vi "Autonomous Independent.vi"   [LabVIEW 2015]
doc: "This VI is called when autonomous begins, and will automatically be terminated when autonomous ends. You can carry out timed or sensor driven robot movement independently without needing to return to the caller."
uses:
  <vilib>/Rock Robotics/WPI/Solenoid/WPI_SolenoidValue.ctl
  <vilib>/Rock Robotics/WPI/Utilities/WPI_GetSetVariantRefNum.vi
  <vilib>/Rock Robotics/Network Tables/NT Write Numeric Array.vi
  <vilib>/Rock Robotics/Network Tables/NT Read String.vi
  <vilib>/Rock Robotics/WPI/Solenoid/WPI_SolenoidSetEnum.vi
  <vilib>/Rock Robotics/WPI/RobotDrive/WPI_RobotDriveArcadeDrive_Standard(NoSaturation).vi
panel:
  # "Be sure to right-click and choose Data Operations>>Make Current Value default if you want to save the array values with the VI"
types:
  T1 = typedef "WPI_JoystickDevRef.ctl" = cluster{"Device":T2}
  T2 = typedef "WPI_JoystickDeviceEnum.ctl" = enum16{"USB 0", "USB 1", "USB 2", "USB 3", "USB 4", "USB 5"}
  T3 = typedef "WPI_SolenoidValue.ctl" = enum16{"Off", "On", "Forward", "Reverse"}
  T4 = typedef "WPI_SolenoidDevRef.ctl" = cluster{"DevStatus":errorcluster, "Pneumatics Control Module":u8, "Forward Solenoid Channel":T5, "Reverse Solenoid Channel":T5}
  T5 = typedef "WPI_SolenoidChannel.ctl" = enum8{"Solenoid 0", "Solenoid 1", "Solenoid 2", "Solenoid 3", "Solenoid 4", "Solenoid 5", "Solenoid 6", "Solenoid 7", "Invalid"}
  T6 = typedef "WPI_RobotDriveDevRef.ctl" = cluster{"DevStatus":errorcluster, "Motors[]":T7[], "Square Inputs":bool, "Max Output":dbl}
  T7 = typedef "WPI_MotorControlDeviceRef.ctl" = cluster{"DeviceStatus":errorcluster, "Type":T8, "PWM":cluster{"PWM Channel":T9, "DeadBand":T10}, "CAN":cluster{"Device Number":u8, "Control Mode":T11, "Semaphore":T12, "Max Vout":dbl, "TalonSRX Control Mode":T13}, "Invert":bool}
  T8 = typedef "WPI_MotorControlType.ctl" = enum16{"PWM", "CAN", "CANTalonSRX"}
  T9 = typedef "FPGA_DIOPWMChannel.ctl" = enum8{"PWM 0", "PWM 1", "PWM 2", "PWM 3", "PWM 4", "PWM 5", "PWM 6", "PWM 7", "PWM 8", "PWM 9", "PWM MXP 0", "PWM MXP 1", "PWM MXP 2", "PWM MXP 3", "PWM MXP 4", "PWM MXP 5", "PWM MXP 6", "PWM MXP 7", "PWM MXP 8", "PWM MXP 9", "Invalid"}
  T10 = typedef "WPI_PWMDeadband.ctl" = cluster{"Name":string, "maxPositivePwm":i32, "minPositivePwm":i32, "centerPwm":i32, "maxNegativePwm":i32, "minNegativePwm":i32, "angularRange":u16}
  T11 = typedef "WPI_CANJaguar_ControlMode.ctl" = enum8{"Percent VBus", "Current", "Speed", "Position", "Voltage"}
  T12 = typedef "Semaphore RefNum" = refnum<k1>
  T13 = typedef "WPI_CANTalonSRX_APIControlMode.ctl" = enum8{"Percent VBus", "Speed", "Position", "Slave", "Unchanged / Invalid", "Voltage Compensation", "Current", "Motion Profile"}
  T14 = typedef "WPI_EncoderDevRef.ctl" = cluster{"DevStatus":errorcluster, "EncoderIndex":T15, "CounterIndex":T16, "DistancePerCount":dbl, "Decoding Type":T17}
  T15 = typedef "FPGA_EncoderIdx.ctl" = enum8{"Enc 0", "Enc 1", "Enc 2", "Enc 3", "Enc 4", "Enc 5", "Enc 6", "Enc 7", "Invalid"}
  T16 = typedef "FPGA_CounterCtrSystemIndex.ctl" = enum8{"Ctr 0", "Ctr 1", "Ctr 2", "Ctr 3", "Ctr 4", "Ctr 5", "Ctr 6", "Ctr 7", "Invalid"}
  T17 = typedef "WPI_EncoderType.ctl" = enum16{"1x", "2x", "4x"}
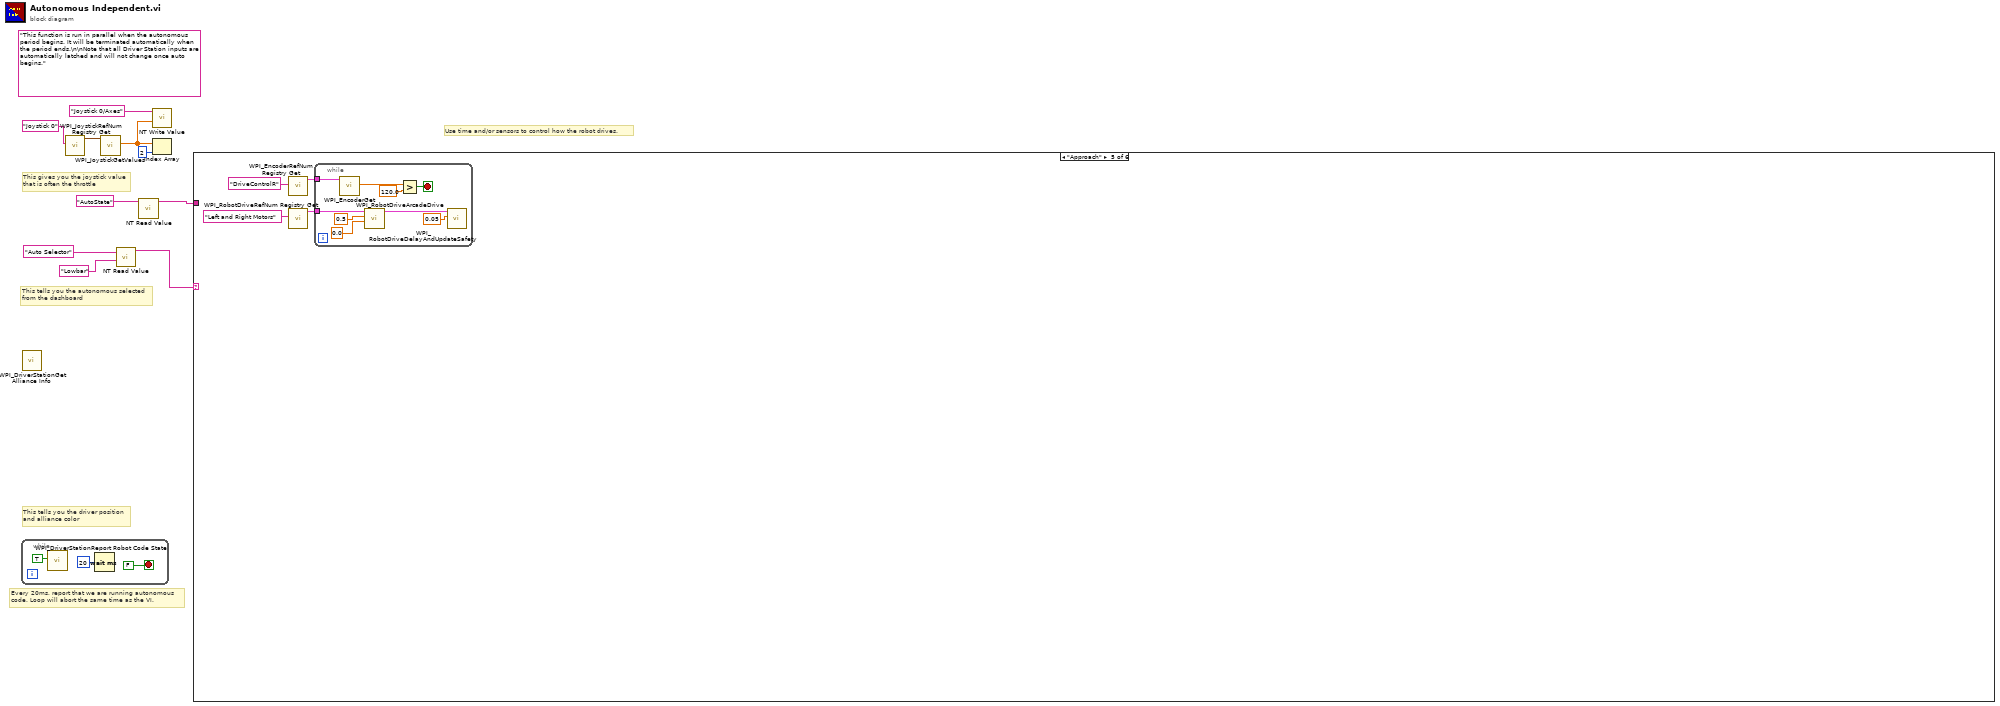
[diagram p0: block diagram]
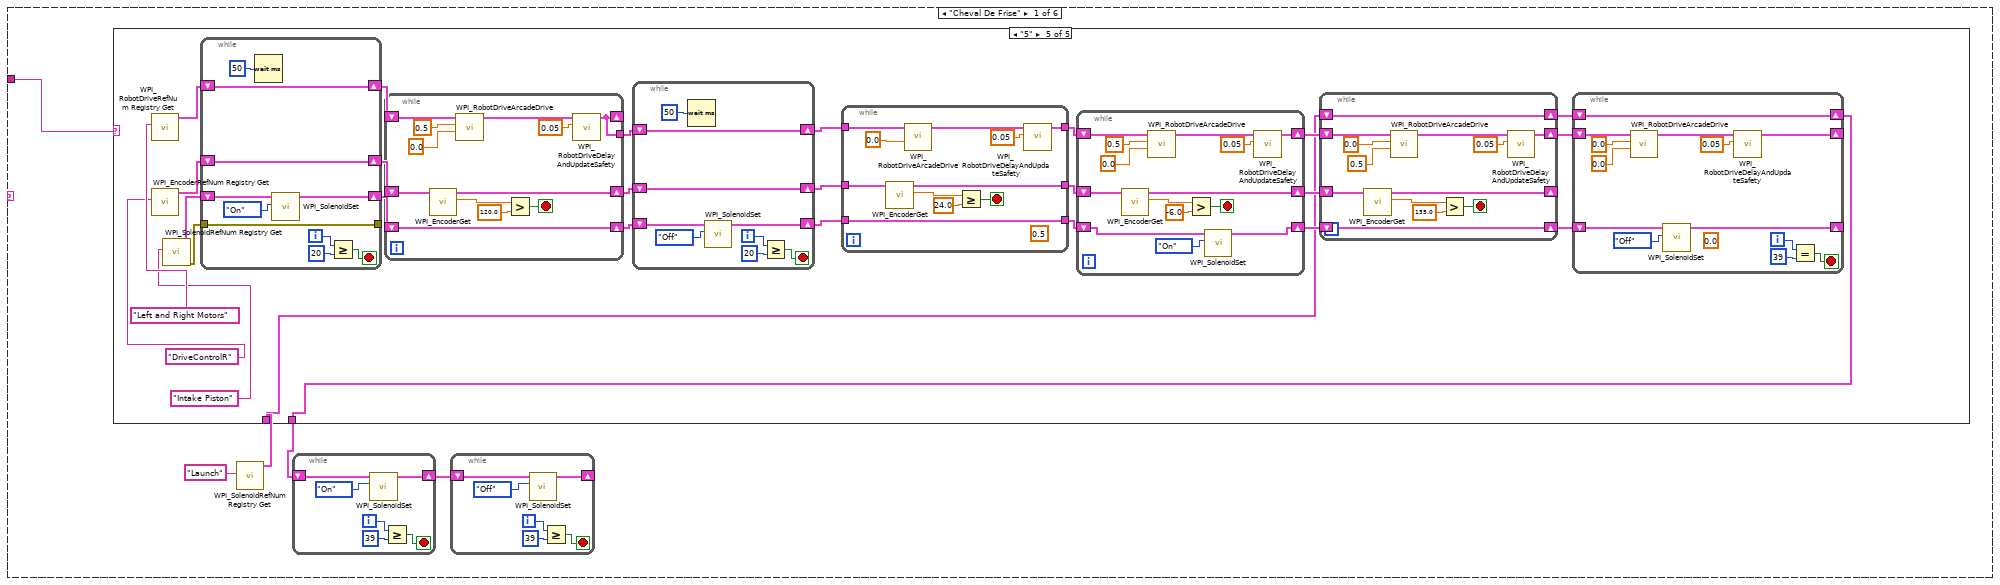
[diagram p2: hidden frame]
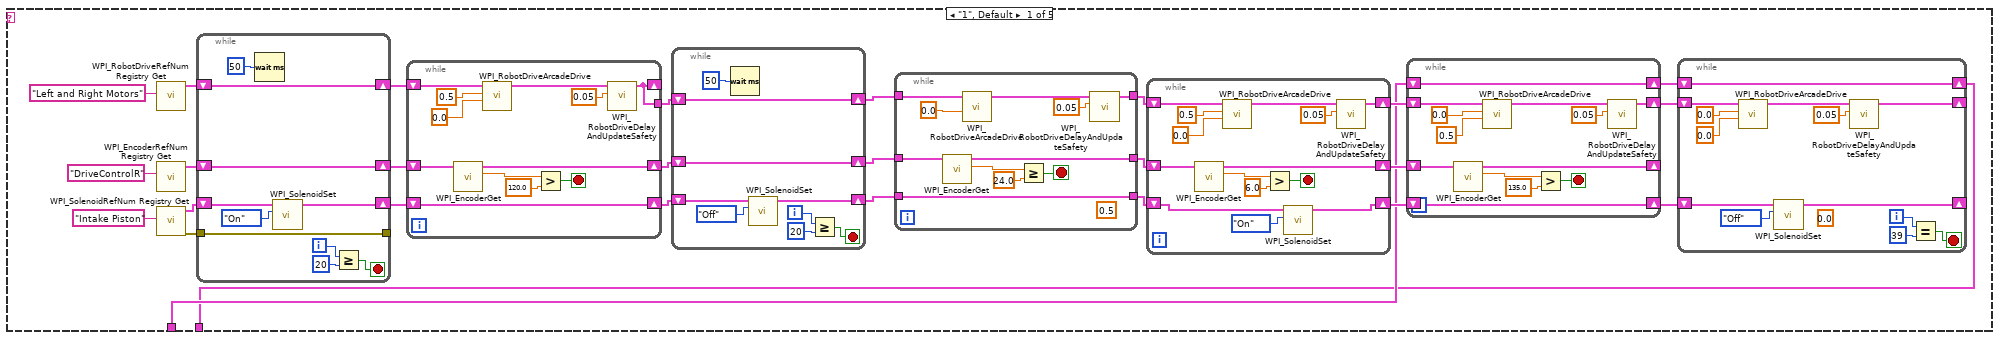
[diagram p3: hidden frame]
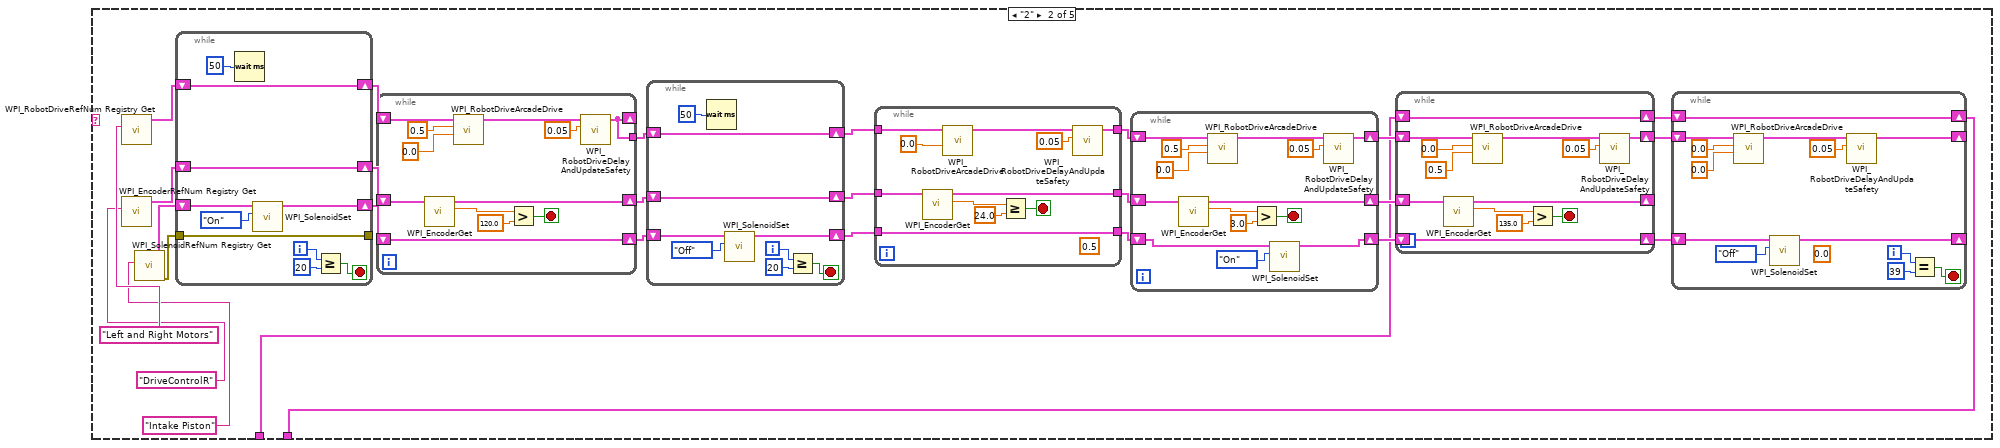
[diagram p4: hidden frame]
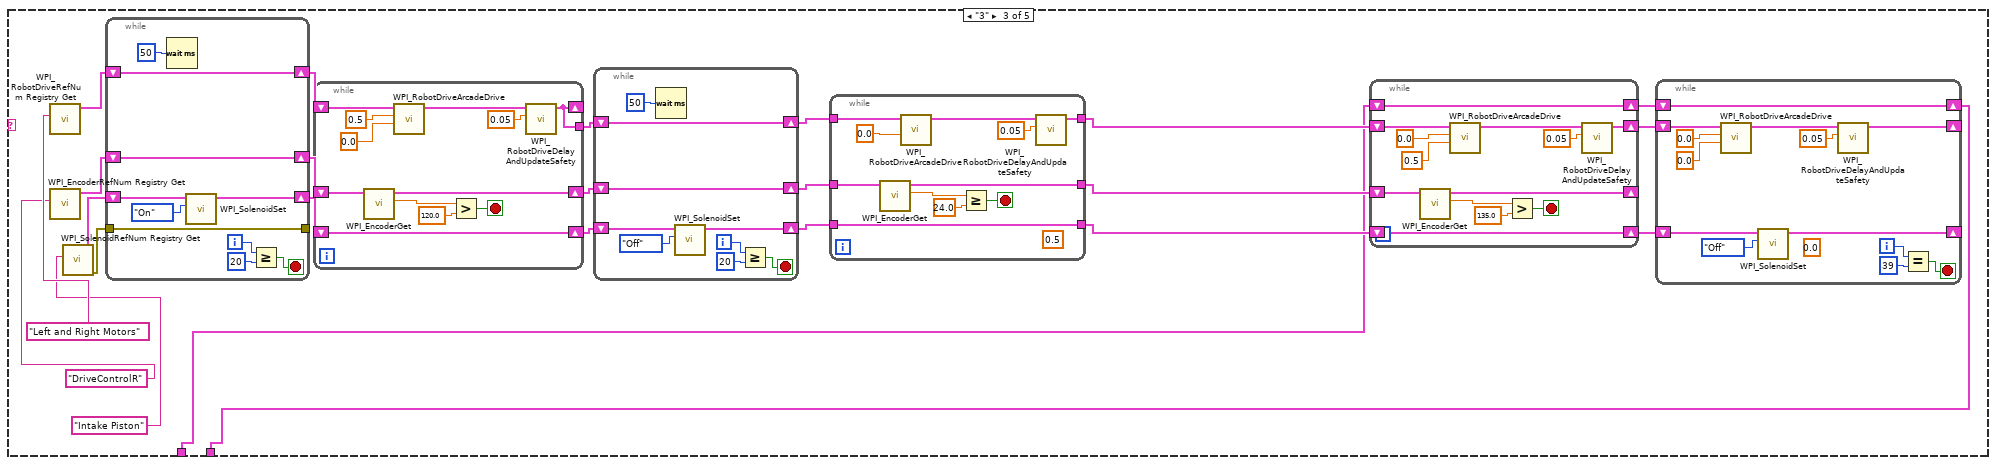
[diagram p5: hidden frame]
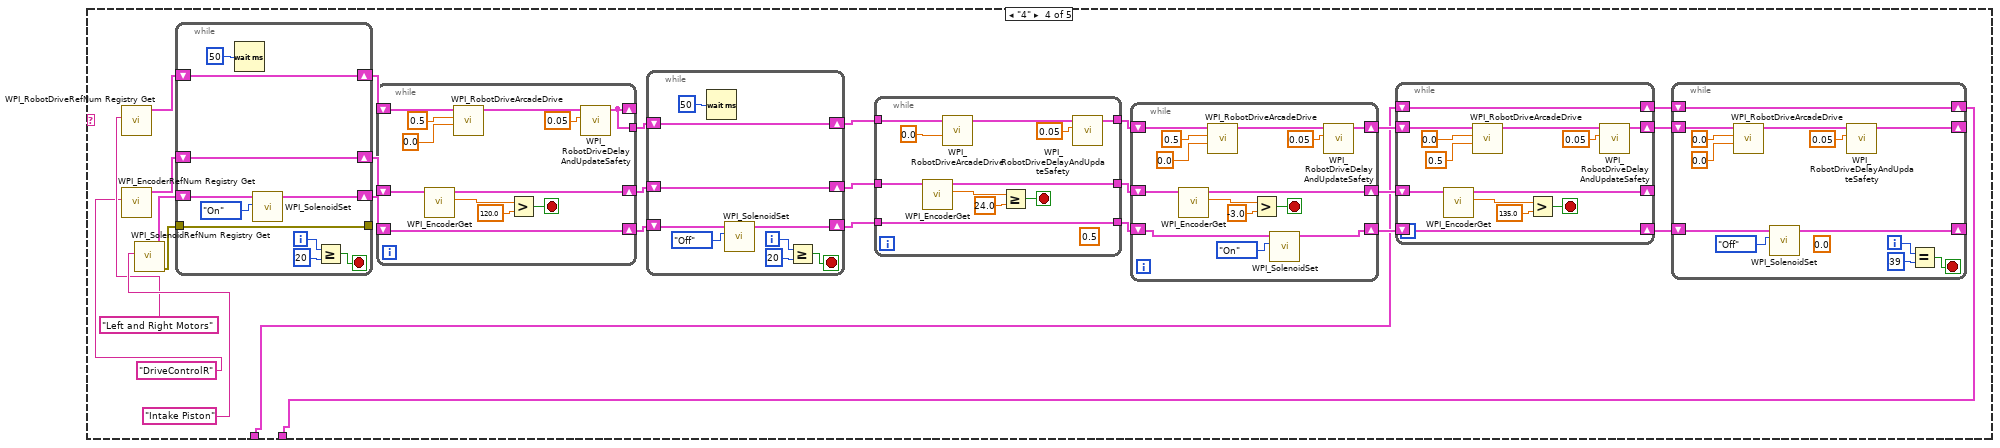
[diagram p6: hidden frame]
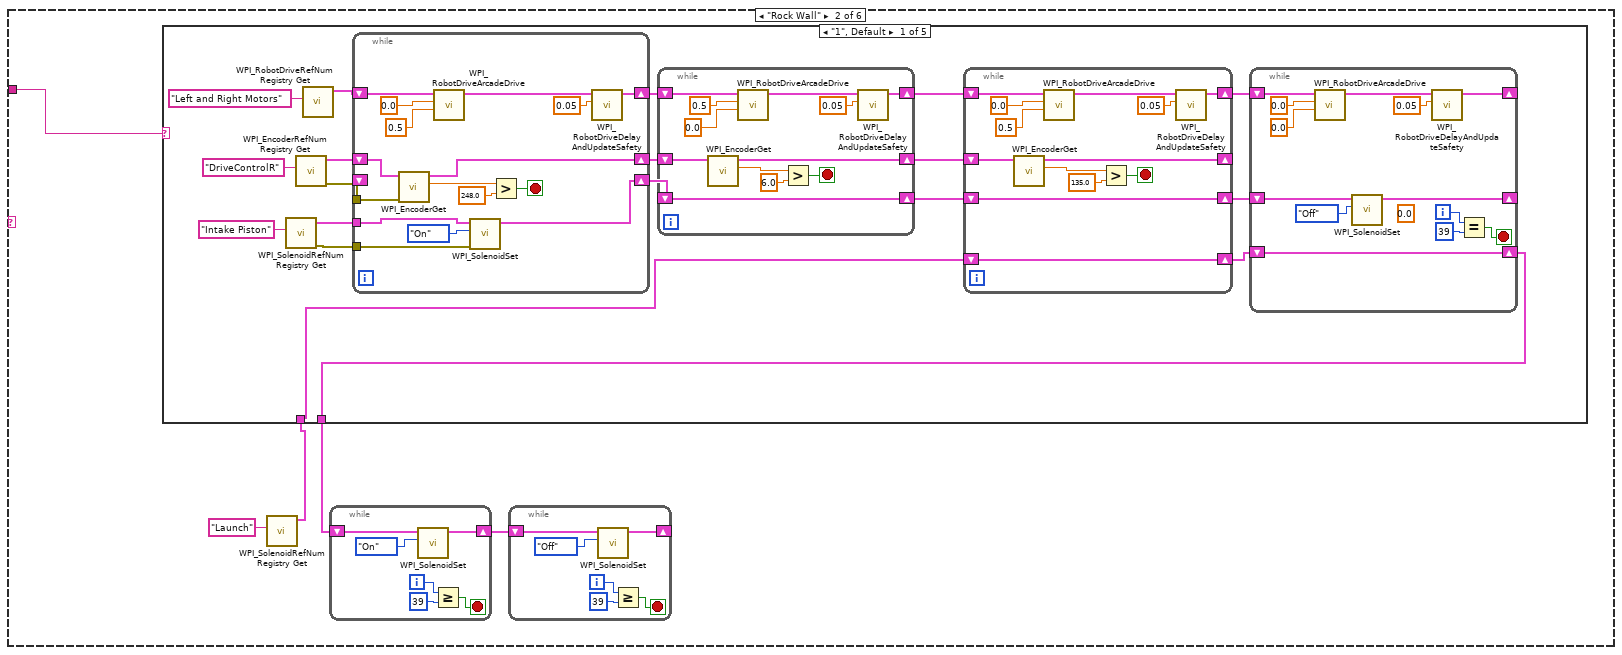
[diagram p7: hidden frame]
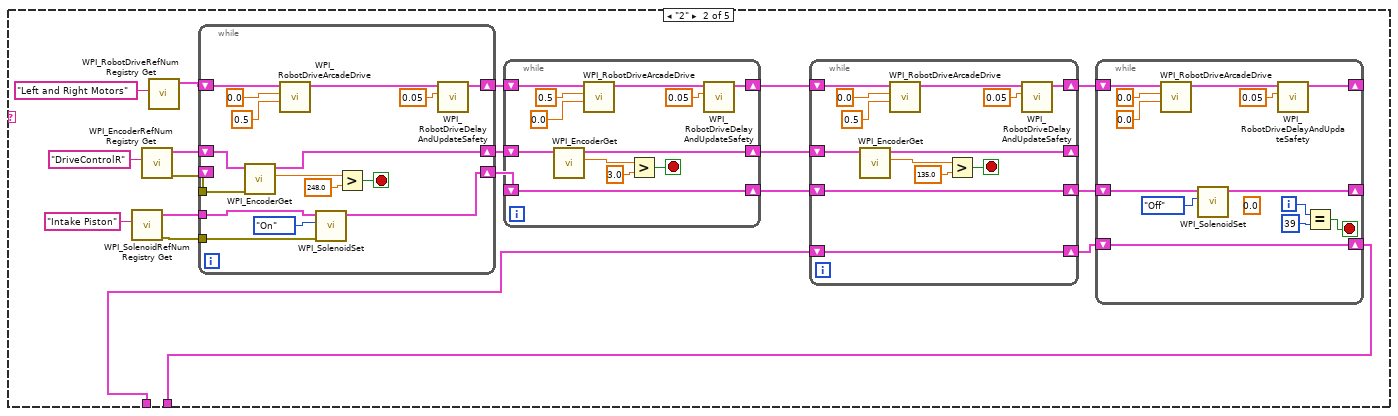
[diagram p8: hidden frame]
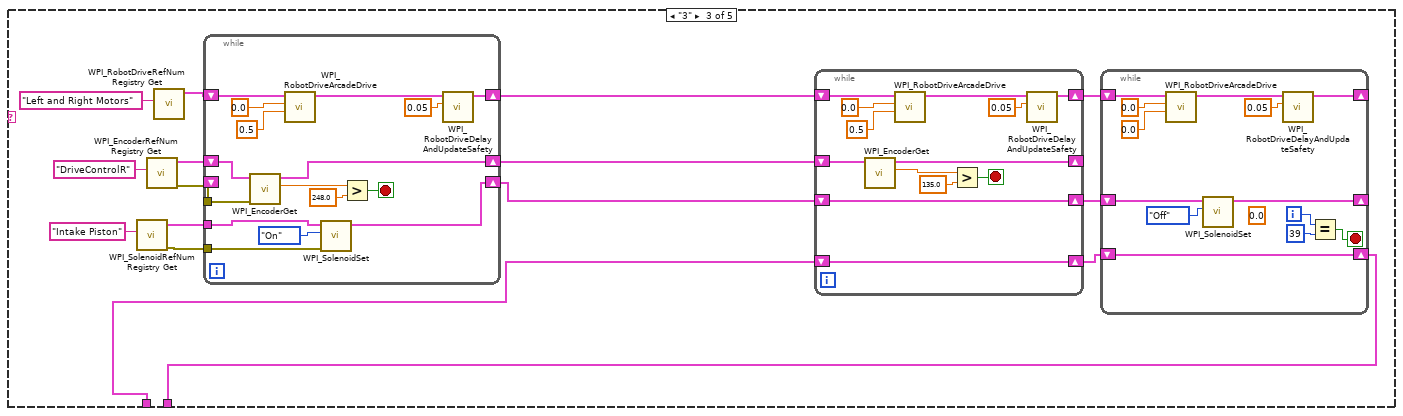
[diagram p9: hidden frame]
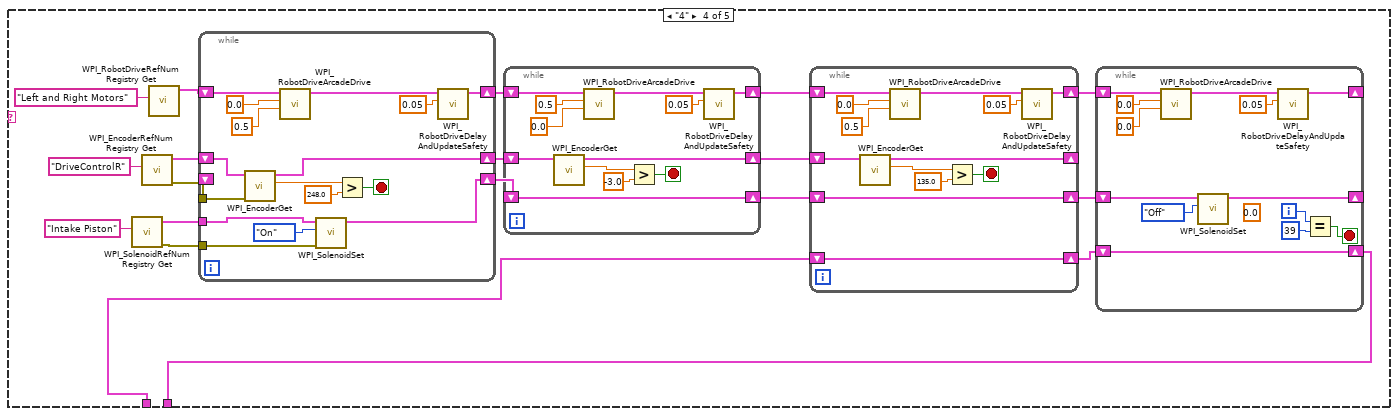
[diagram p10: hidden frame]
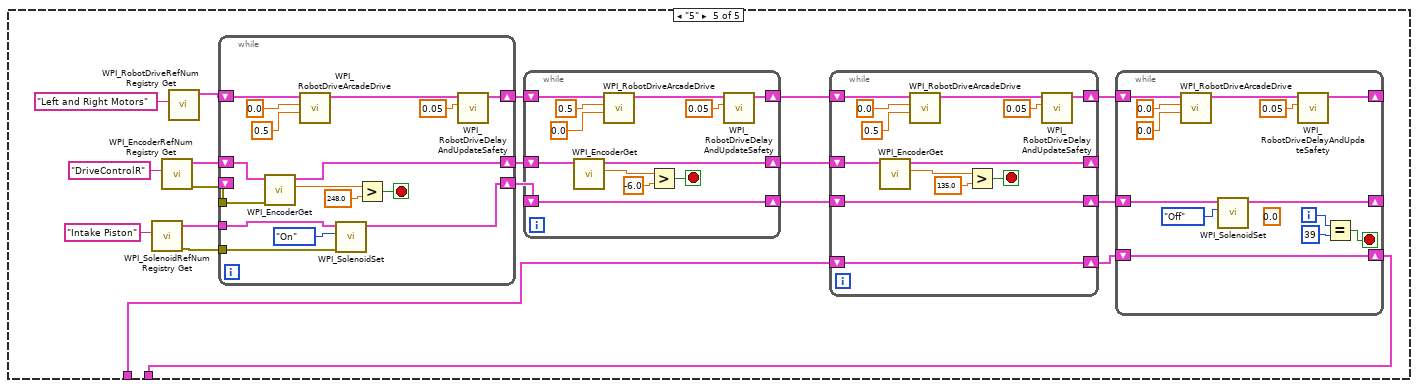
[diagram p11: hidden frame]
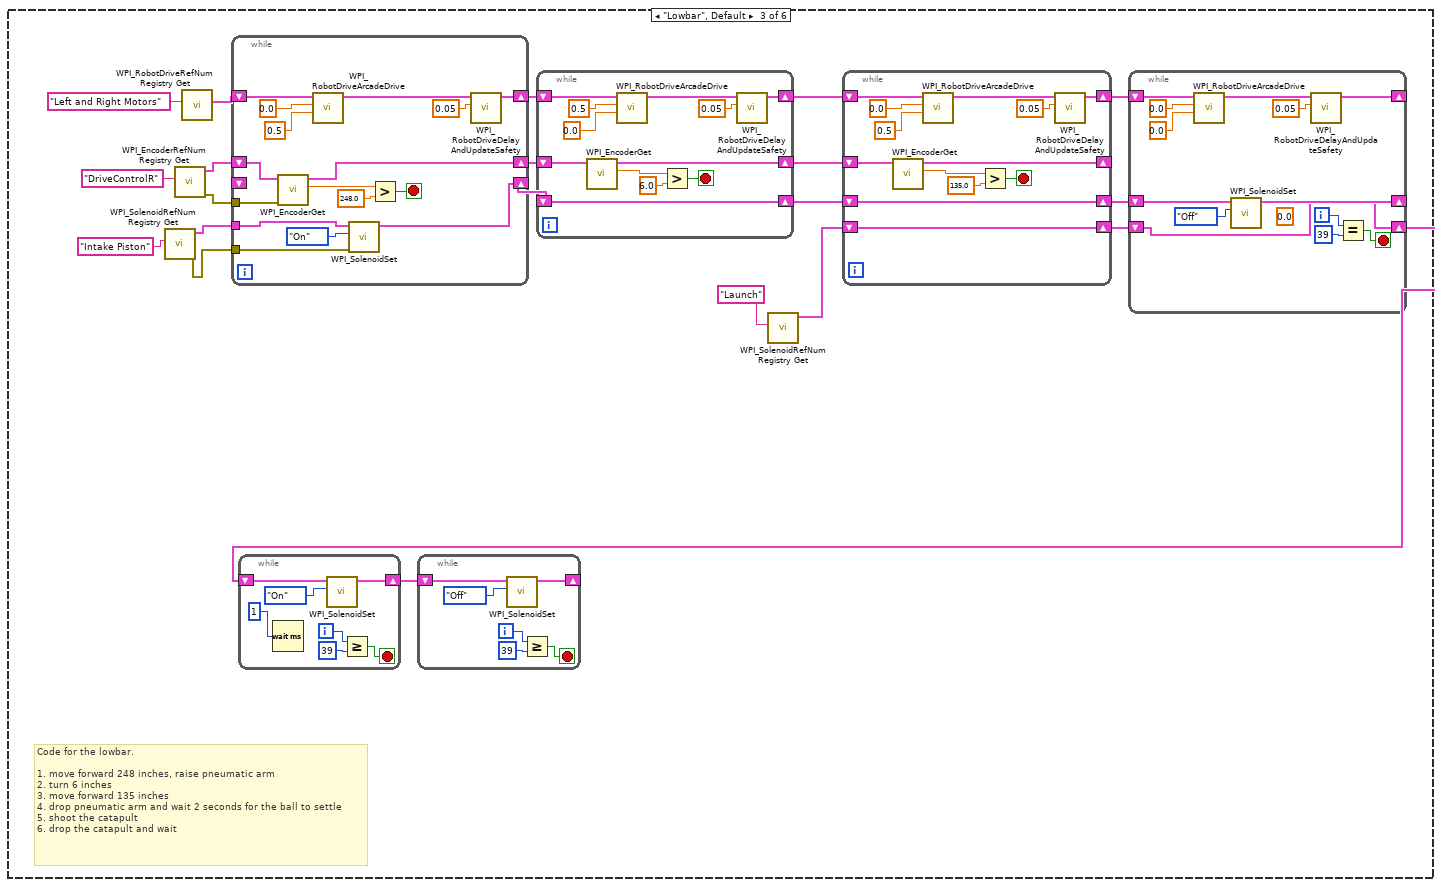
[diagram p12: hidden frame]
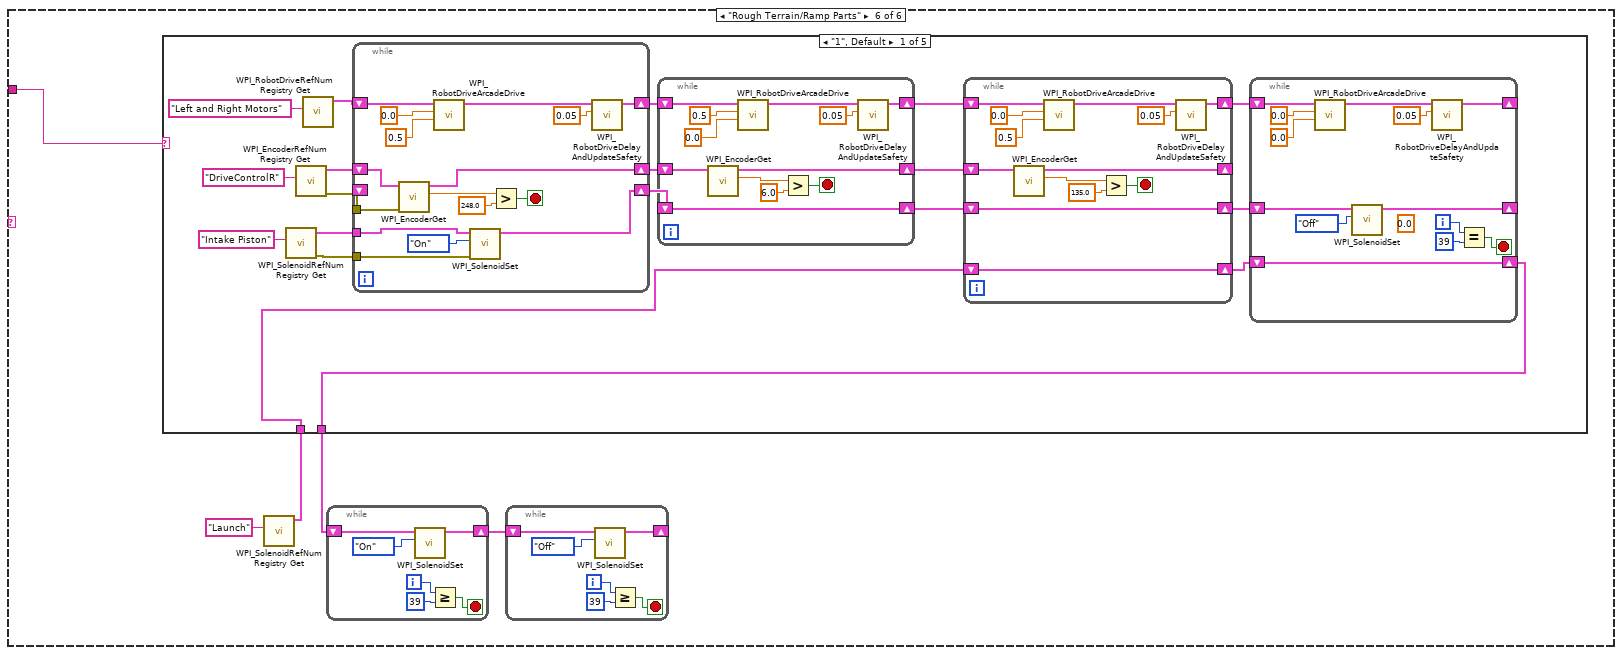
[diagram p14: hidden frame]
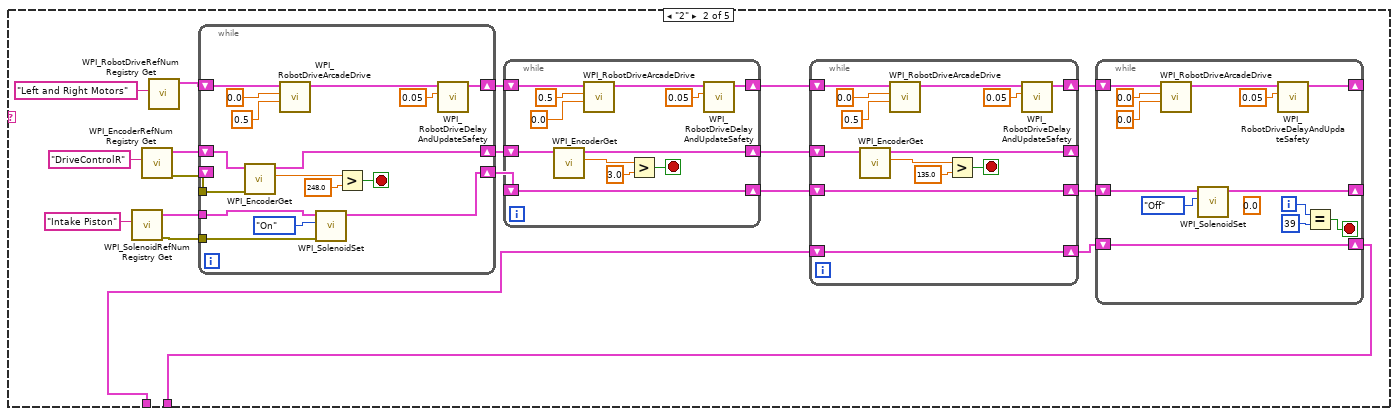
[diagram p15: hidden frame]
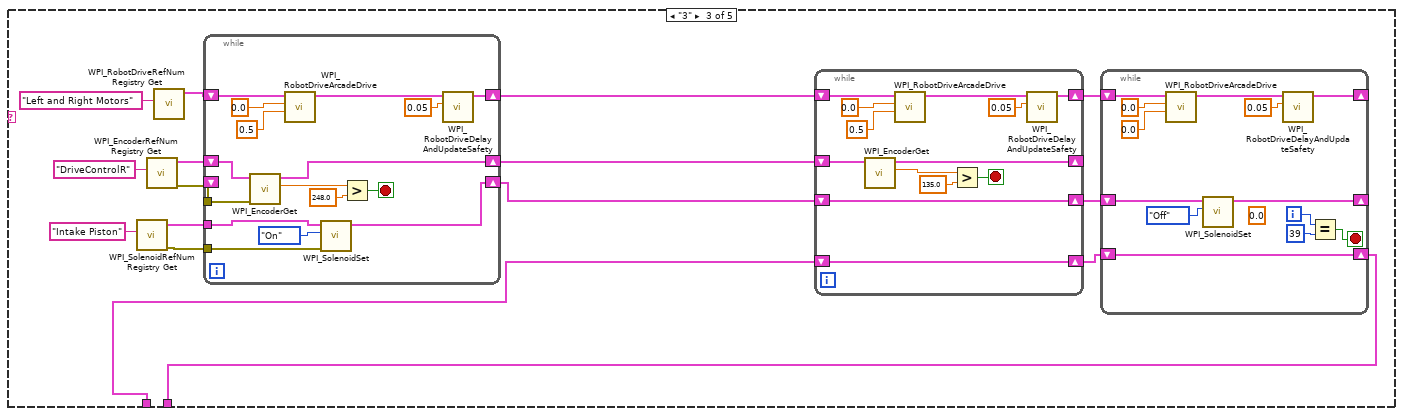
[diagram p16: hidden frame]
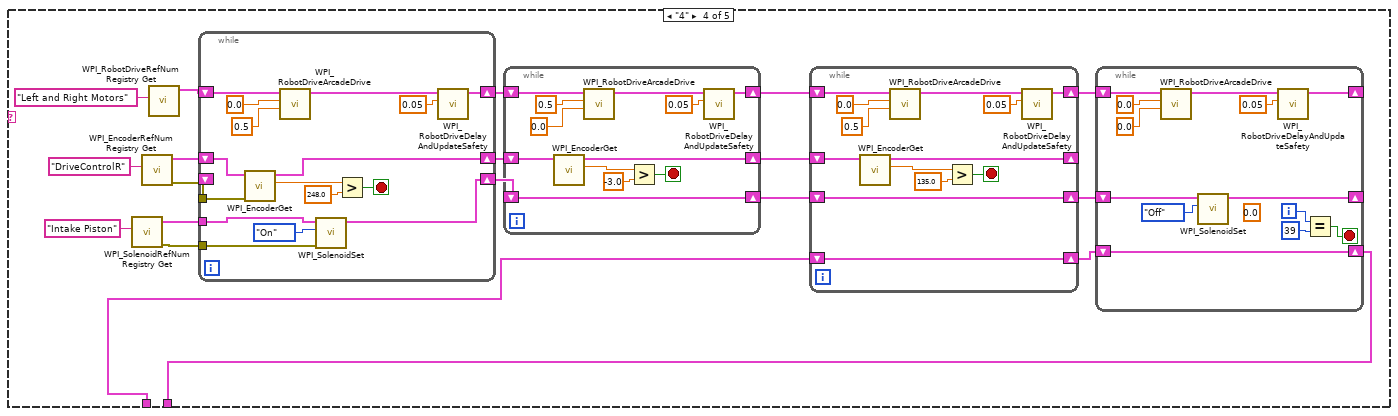
[diagram p17: hidden frame]
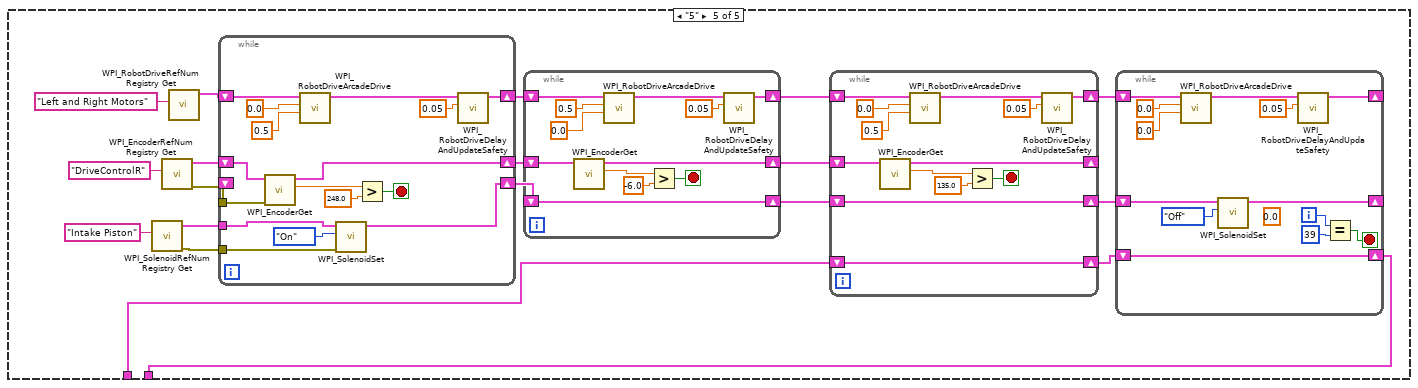
[diagram p18: hidden frame]
diagram:
  (unwired) "This function is run in parallel when the autonomous period begins. It will be terminated automatically when the period ends.\n\nNote that all Driver Station inputs are automatically latched and will not change once auto begins."
  # "This tells you the autonomous selected\nfrom the dashboard"
  # "Every 20ms, report that we are running autonomous\ncode. Loop will abort the same time as the VI."
  # "This gives you the joystick value\nthat is often the throttle"
  # "Use time and/or sensors to control how the robot drives."
  # "This tells you the driver position\nand alliance color"
  n1 = while {
    stop <- FALSE stop-if-true
    n2 = call <vilib>:"WPI_DriverStationReport Robot Code State.vi"("Autonomous"=TRUE) -> ()  [unwired: 10 in, 1 out]
    n3 = Wait (ms)(milliseconds to wait=u32 20) -> ()  [unwired: 1 out]
  }
  n4 = call <vilib>:"WPI_DriverStationGet Alliance Info.vi"() -> ()  [unwired: 12 out]
  n5 = call <vilib>:"WPI_JoystickRefNum Registry Get.vi"("refnum name"="Joystick 0") -> ("JoystickDevRef"=w9:T1)  [unwired: 1 in, 9 out]
  n6 = call <vilib>:"WPI_JoystickGetValues.vi"("JoystickDevRef"=w9) -> ("Axes"=w6:dbl[])  [unwired: 6 in, 4 out]
  n7 = call-poly <vilib>:"NT Read Value.vi"("Default Value"="Lowbar", "Name"="Auto Selector") -> ("String"=w4:string)  [unwired: 8 in, 1 out]
  n8 = call-poly <vilib>:"NT Read Value.vi"("Name"="AutoState") -> ("String"=w2:string)  [unwired: 9 in, 1 out]
  n9 = call-poly <vilib>:"NT Write Value.vi"("Numeric Array"=w6, "Name"="Joystick 0/Axes") -> ()  [unwired: 9 in, 1 out]
  n10 = Index Array(array=w6, index=2) -> ()  [unwired: 1 out]
  n11 = case shown="\"Approach\"" w4 {
    tunnel: w2 -> [w15 w559 _ _ _ w1027]
    frame "Cheval De Frise" {
      n12 = call <vilib>:"WPI_SolenoidRefNum Registry Get.vi"("refnum name"="Launch") -> ("SolenoidDevRef"=w16:T4)  [unwired: 9 in, 1 out]
      n13 = case shown="\"5\"" w15 {
        tunnel: w16 -> [w37 w132 w239 w330 w440]
        tunnel: [w36 w131 w238 w331 w439] -> w14
        frame "1", Default {
          n14 = call <vilib>:"WPI_RobotDriveRefNum Registry Get.vi"("refnum name"="Left and Right Motors") -> ("RobotDriveDevRef"=w31:T6)  [unwired: 1 in, 9 out]
          n15 = call <vilib>:"WPI_EncoderRefNum Registry Get.vi"("refnum name"="DriveControlR") -> ("EncoderDevRef"=w33:T14)  [unwired: 9 in, 1 out]
          n16 = call <vilib>:"WPI_SolenoidRefNum Registry Get.vi"("refnum name"="Intake Piston") -> ("error out"=w34:errorcluster, "SolenoidDevRef"=w35:T4)  [unwired: 9 in]
          n17 = while {
            tunnel: w34 -> [w87]
            tunnel: [w87] -> _
            shift-right: [w83] -> w28
            shift-left: w35 -> [w84]
            shift-right: [w86] -> w30
            shift-left: w33 -> [w86]
            shift-right: [w78] -> w32
            shift-left: w31 -> [w78]
            i -> [w81]
            stop <- w82 stop-if-true
            n18 = Wait (ms)(milliseconds to wait=u32 50) -> ()  [unwired: 1 out]
            n19 = call-poly <vilib>:"WPI_SolenoidSet.vi"("Value"=WPI_SolenoidValue."On", "SolenoidDevRef"=w84) -> ("SolenoidDevRef"=w83:T4)  [unwired: 8 in, 1 out]
            n20 = Greater Or Equal?(x=w81, y=20) -> (x >= y?=w82:bool)
          }
          n21 = while {
            shift-right: [w66] -> _
            shift-left: w32 -> [w73]
            shift-right: [w69] -> w23
            shift-left: w30 -> [w70]
            shift-right: [w67] -> w24
            shift-left: w28 -> [w67]
            tunnel: [w66] -> w22
            stop <- w72 stop-if-true
            n22 = call <vilib>:"WPI_EncoderGet.vi"("EncoderDevRef"=w70) -> ("Distance"=w71:dbl, "EncoderDevRef"=w69:T14)  [unwired: 5 in, 4 out]
            n23 = call-poly <vilib>:"WPI_RobotDriveArcadeDrive.vi"("Y axis value"=0.0 ("X axis value"), "X axis value"=0.5, "RobotDriveDevRef"=w73) -> ("RobotDriveDevRef"=w75:T6)  [unwired: 1 in, 7 out]
            n24 = Greater?(x=w71, y=120.0) -> (0:w72:bool)
            n25 = call <vilib>:"WPI_RobotDriveDelayAndUpdateSafety.vi"("Delay (s)"=0.05, "RobotDriveDevRef"=w75) -> ("RobotDriveDevRef 2"=w66:T6)  [unwired: 8 in, 1 out]
          }
          n26 = while {
            shift-right: [w60] -> w25
            shift-left: w24 -> [w59]
            shift-right: [w58] -> w26
            shift-left: w23 -> [w58]
            shift-right: [w57] -> w27
            shift-left: w22 -> [w57]
            i -> [w64]
            stop <- w65 stop-if-true
            n27 = Wait (ms)(milliseconds to wait=u32 50) -> ()  [unwired: 1 out]
            n28 = call-poly <vilib>:"WPI_SolenoidSet.vi"("Value"=WPI_SolenoidValue."Off", "SolenoidDevRef"=w59) -> ("SolenoidDevRef"=w60:T4)  [unwired: 8 in, 1 out]
            n29 = Greater Or Equal?(x=w64, y=20) -> (x >= y?=w65:bool)
          }
          n30 = while {
            tunnel: [w50] -> w21
            tunnel: w27 -> [w49]
            tunnel: w26 -> [w48]
            tunnel: [w47] -> w20
            tunnel: w25 -> [w46]
            tunnel: [w46] -> w19
            stop <- w56 stop-if-true
            (unwired) 0.5 ("X axis value")
            n31 = call <vilib>:"WPI_EncoderGet.vi"("EncoderDevRef"=w48) -> ("Distance"=w55:dbl, "EncoderDevRef"=w47:T14)  [unwired: 5 in, 4 out]
            n32 = call-poly <vilib>:"WPI_RobotDriveArcadeDrive.vi"("Y axis value"=0.0 ("X axis value"), "RobotDriveDevRef"=w49) -> ("RobotDriveDevRef"=w52:T6)  [unwired: 2 in, 7 out]
            n33 = Greater Or Equal?(x=w55, y=24.0) -> (x >= y?=w56:bool)
            n34 = call <vilib>:"WPI_RobotDriveDelayAndUpdateSafety.vi"("Delay (s)"=0.05, "RobotDriveDevRef"=w52) -> ("RobotDriveDevRef 2"=w50:T6)  [unwired: 8 in, 1 out]
          }
          n35 = while {
            shift-right: [w126] -> w42
            shift-left: w21 -> [w118]
            shift-right: [w114] -> w40
            shift-left: w19 -> [w115]
            shift-right: [w117] -> w41
            shift-left: w20 -> [w119]
            stop <- w120 stop-if-true
            n36 = call <vilib>:"WPI_EncoderGet.vi"("EncoderDevRef"=w119) -> ("Distance"=w121:dbl, "EncoderDevRef"=w117:T14)  [unwired: 5 in, 4 out]
            n37 = call-poly <vilib>:"WPI_RobotDriveArcadeDrive.vi"("Y axis value"=0.0 ("X axis value"), "X axis value"=0.5, "RobotDriveDevRef"=w118) -> ("RobotDriveDevRef"=w125:T6)  [unwired: 1 in, 7 out]
            n38 = Greater?(x=w121, y=6.0) -> (0:w120:bool)
            n39 = call-poly <vilib>:"WPI_SolenoidSet.vi"("Value"=WPI_SolenoidValue."On", "SolenoidDevRef"=w115) -> ("SolenoidDevRef"=w114:T4)  [unwired: 8 in, 1 out]
            n40 = call <vilib>:"WPI_RobotDriveDelayAndUpdateSafety.vi"("Delay (s)"=0.05, "RobotDriveDevRef"=w125) -> ("RobotDriveDevRef 2"=w126:T6)  [unwired: 8 in, 1 out]
          }
          n41 = while {
            shift-right: [w105] -> w39
            shift-left: w42 -> [w108]
            shift-right: [w103] -> w29
            shift-left: w40 -> [w103]
            shift-right: [w102] -> _
            shift-left: w41 -> [w104]
            shift-right: [w101] -> w38
            shift-left: w37 -> [w101]
            stop <- w111 stop-if-true
            n42 = call <vilib>:"WPI_EncoderGet.vi"("EncoderDevRef"=w104) -> ("Distance"=w112:dbl, "EncoderDevRef"=w102:T14)  [unwired: 5 in, 4 out]
            n43 = call-poly <vilib>:"WPI_RobotDriveArcadeDrive.vi"("Y axis value"=0.5 ("X axis value"), "X axis value"=0.0, "RobotDriveDevRef"=w108) -> ("RobotDriveDevRef"=w107:T6)  [unwired: 1 in, 7 out]
            n44 = Greater?(x=w112, y=135.0) -> (0:w111:bool)
            n45 = call <vilib>:"WPI_RobotDriveDelayAndUpdateSafety.vi"("Delay (s)"=0.05, "RobotDriveDevRef"=w107) -> ("RobotDriveDevRef 2"=w105:T6)  [unwired: 8 in, 1 out]
          }
          n46 = while {
            shift-right: [w94] -> _
            shift-left: w39 -> [w98]
            shift-right: [w88] -> _
            shift-left: w29 -> [w89]
            shift-right: [w90] -> w36
            shift-left: w38 -> [w90]
            i -> [w93]
            stop <- w91 stop-if-true
            (unwired) 0.0 ("Set Start Time (s)")
            n47 = call-poly <vilib>:"WPI_RobotDriveArcadeDrive.vi"("Y axis value"=0.0, "X axis value"=0.0, "RobotDriveDevRef"=w98) -> ("RobotDriveDevRef"=w95:T6)  [unwired: 1 in, 7 out]
            n48 = call-poly <vilib>:"WPI_SolenoidSet.vi"("Value"=WPI_SolenoidValue."Off", "SolenoidDevRef"=w89) -> ("SolenoidDevRef"=w88:T4)  [unwired: 8 in, 1 out]
            n49 = call <vilib>:"WPI_RobotDriveDelayAndUpdateSafety.vi"("Delay (s)"=0.05, "RobotDriveDevRef"=w95) -> ("RobotDriveDevRef 2"=w94:T6)  [unwired: 8 in, 1 out]
            n50 = Equal?(x=w93, y=39) -> (x = y?=w91:bool)
          }
        }
        frame "2" {
          n51 = call <vilib>:"WPI_RobotDriveRefNum Registry Get.vi"("refnum name"="Left and Right Motors") -> ("RobotDriveDevRef"=w145:T6)  [unwired: 1 in, 9 out]
          n52 = call <vilib>:"WPI_EncoderRefNum Registry Get.vi"("refnum name"="DriveControlR") -> ("EncoderDevRef"=w147:T14)  [unwired: 9 in, 1 out]
          n53 = call <vilib>:"WPI_SolenoidRefNum Registry Get.vi"("refnum name"="Intake Piston") -> ("error out"=w148:errorcluster, "SolenoidDevRef"=w149:T4)  [unwired: 9 in]
          n54 = while {
            tunnel: w148 -> [w196]
            tunnel: [w196] -> _
            shift-right: [w192] -> w142
            shift-left: w149 -> [w193]
            shift-right: [w195] -> w144
            shift-left: w147 -> [w195]
            shift-right: [w187] -> w146
            shift-left: w145 -> [w187]
            i -> [w190]
            stop <- w191 stop-if-true
            n55 = Wait (ms)(milliseconds to wait=u32 50) -> ()  [unwired: 1 out]
            n56 = call-poly <vilib>:"WPI_SolenoidSet.vi"("Value"=WPI_SolenoidValue."On", "SolenoidDevRef"=w193) -> ("SolenoidDevRef"=w192:T4)  [unwired: 8 in, 1 out]
            n57 = Greater Or Equal?(x=w190, y=20) -> (x >= y?=w191:bool)
          }
          n58 = while {
            shift-right: [w175] -> _
            shift-left: w146 -> [w182]
            shift-right: [w178] -> w137
            shift-left: w144 -> [w179]
            shift-right: [w176] -> w138
            shift-left: w142 -> [w176]
            tunnel: [w175] -> w136
            stop <- w181 stop-if-true
            n59 = call <vilib>:"WPI_EncoderGet.vi"("EncoderDevRef"=w179) -> ("Distance"=w180:dbl, "EncoderDevRef"=w178:T14)  [unwired: 5 in, 4 out]
            n60 = call-poly <vilib>:"WPI_RobotDriveArcadeDrive.vi"("Y axis value"=0.0 ("X axis value"), "X axis value"=0.5, "RobotDriveDevRef"=w182) -> ("RobotDriveDevRef"=w184:T6)  [unwired: 1 in, 7 out]
            n61 = Greater?(x=w180, y=120.0) -> (0:w181:bool)
            n62 = call <vilib>:"WPI_RobotDriveDelayAndUpdateSafety.vi"("Delay (s)"=0.05, "RobotDriveDevRef"=w184) -> ("RobotDriveDevRef 2"=w175:T6)  [unwired: 8 in, 1 out]
          }
          n63 = while {
            shift-right: [w169] -> w139
            shift-left: w138 -> [w168]
            shift-right: [w167] -> w140
            shift-left: w137 -> [w167]
            shift-right: [w166] -> w141
            shift-left: w136 -> [w166]
            i -> [w173]
            stop <- w174 stop-if-true
            n64 = Wait (ms)(milliseconds to wait=u32 50) -> ()  [unwired: 1 out]
            n65 = call-poly <vilib>:"WPI_SolenoidSet.vi"("Value"=WPI_SolenoidValue."Off", "SolenoidDevRef"=w168) -> ("SolenoidDevRef"=w169:T4)  [unwired: 8 in, 1 out]
            n66 = Greater Or Equal?(x=w173, y=20) -> (x >= y?=w174:bool)
          }
          n67 = while {
            tunnel: [w159] -> w135
            tunnel: w141 -> [w158]
            tunnel: w140 -> [w157]
            tunnel: [w156] -> w134
            tunnel: w139 -> [w155]
            tunnel: [w155] -> w133
            stop <- w165 stop-if-true
            (unwired) 0.5 ("X axis value")
            n68 = call <vilib>:"WPI_EncoderGet.vi"("EncoderDevRef"=w157) -> ("Distance"=w164:dbl, "EncoderDevRef"=w156:T14)  [unwired: 5 in, 4 out]
            n69 = call-poly <vilib>:"WPI_RobotDriveArcadeDrive.vi"("Y axis value"=0.0 ("X axis value"), "RobotDriveDevRef"=w158) -> ("RobotDriveDevRef"=w161:T6)  [unwired: 2 in, 7 out]
            n70 = Greater Or Equal?(x=w164, y=24.0) -> (x >= y?=w165:bool)
            n71 = call <vilib>:"WPI_RobotDriveDelayAndUpdateSafety.vi"("Delay (s)"=0.05, "RobotDriveDevRef"=w161) -> ("RobotDriveDevRef 2"=w159:T6)  [unwired: 8 in, 1 out]
          }
          n72 = while {
            shift-right: [w235] -> w154
            shift-left: w135 -> [w227]
            shift-right: [w223] -> w152
            shift-left: w133 -> [w224]
            shift-right: [w226] -> w153
            shift-left: w134 -> [w228]
            stop <- w229 stop-if-true
            n73 = call <vilib>:"WPI_EncoderGet.vi"("EncoderDevRef"=w228) -> ("Distance"=w230:dbl, "EncoderDevRef"=w226:T14)  [unwired: 5 in, 4 out]
            n74 = call-poly <vilib>:"WPI_RobotDriveArcadeDrive.vi"("Y axis value"=0.0 ("X axis value"), "X axis value"=0.5, "RobotDriveDevRef"=w227) -> ("RobotDriveDevRef"=w234:T6)  [unwired: 1 in, 7 out]
            n75 = Greater?(x=w230, y=3.0) -> (0:w229:bool)
            n76 = call-poly <vilib>:"WPI_SolenoidSet.vi"("Value"=WPI_SolenoidValue."On", "SolenoidDevRef"=w224) -> ("SolenoidDevRef"=w223:T4)  [unwired: 8 in, 1 out]
            n77 = call <vilib>:"WPI_RobotDriveDelayAndUpdateSafety.vi"("Delay (s)"=0.05, "RobotDriveDevRef"=w234) -> ("RobotDriveDevRef 2"=w235:T6)  [unwired: 8 in, 1 out]
          }
          n78 = while {
            shift-right: [w214] -> w151
            shift-left: w154 -> [w217]
            shift-right: [w212] -> w143
            shift-left: w152 -> [w212]
            shift-right: [w211] -> _
            shift-left: w153 -> [w213]
            shift-right: [w210] -> w150
            shift-left: w132 -> [w210]
            stop <- w220 stop-if-true
            n79 = call <vilib>:"WPI_EncoderGet.vi"("EncoderDevRef"=w213) -> ("Distance"=w221:dbl, "EncoderDevRef"=w211:T14)  [unwired: 5 in, 4 out]
            n80 = call-poly <vilib>:"WPI_RobotDriveArcadeDrive.vi"("Y axis value"=0.5 ("X axis value"), "X axis value"=0.0, "RobotDriveDevRef"=w217) -> ("RobotDriveDevRef"=w216:T6)  [unwired: 1 in, 7 out]
            n81 = Greater?(x=w221, y=135.0) -> (0:w220:bool)
            n82 = call <vilib>:"WPI_RobotDriveDelayAndUpdateSafety.vi"("Delay (s)"=0.05, "RobotDriveDevRef"=w216) -> ("RobotDriveDevRef 2"=w214:T6)  [unwired: 8 in, 1 out]
          }
          n83 = while {
            shift-right: [w203] -> _
            shift-left: w151 -> [w207]
            shift-right: [w197] -> _
            shift-left: w143 -> [w198]
            shift-right: [w199] -> w131
            shift-left: w150 -> [w199]
            i -> [w202]
            stop <- w200 stop-if-true
            (unwired) 0.0 ("Set Start Time (s)")
            n84 = call-poly <vilib>:"WPI_RobotDriveArcadeDrive.vi"("Y axis value"=0.0, "X axis value"=0.0, "RobotDriveDevRef"=w207) -> ("RobotDriveDevRef"=w204:T6)  [unwired: 1 in, 7 out]
            n85 = call-poly <vilib>:"WPI_SolenoidSet.vi"("Value"=WPI_SolenoidValue."Off", "SolenoidDevRef"=w198) -> ("SolenoidDevRef"=w197:T4)  [unwired: 8 in, 1 out]
            n86 = call <vilib>:"WPI_RobotDriveDelayAndUpdateSafety.vi"("Delay (s)"=0.05, "RobotDriveDevRef"=w204) -> ("RobotDriveDevRef 2"=w203:T6)  [unwired: 8 in, 1 out]
            n87 = Equal?(x=w202, y=39) -> (x = y?=w200:bool)
          }
        }
        frame "3" {
          n88 = call <vilib>:"WPI_RobotDriveRefNum Registry Get.vi"("refnum name"="Left and Right Motors") -> ("RobotDriveDevRef"=w251:T6)  [unwired: 1 in, 9 out]
          n89 = call <vilib>:"WPI_EncoderRefNum Registry Get.vi"("refnum name"="DriveControlR") -> ("EncoderDevRef"=w253:T14)  [unwired: 9 in, 1 out]
          n90 = call <vilib>:"WPI_SolenoidRefNum Registry Get.vi"("refnum name"="Intake Piston") -> ("error out"=w254:errorcluster, "SolenoidDevRef"=w255:T4)  [unwired: 9 in]
          n91 = while {
            tunnel: w254 -> [w302]
            tunnel: [w302] -> _
            shift-right: [w298] -> w248
            shift-left: w255 -> [w299]
            shift-right: [w301] -> w250
            shift-left: w253 -> [w301]
            shift-right: [w293] -> w252
            shift-left: w251 -> [w293]
            i -> [w296]
            stop <- w297 stop-if-true
            n92 = Wait (ms)(milliseconds to wait=u32 50) -> ()  [unwired: 1 out]
            n93 = call-poly <vilib>:"WPI_SolenoidSet.vi"("Value"=WPI_SolenoidValue."On", "SolenoidDevRef"=w299) -> ("SolenoidDevRef"=w298:T4)  [unwired: 8 in, 1 out]
            n94 = Greater Or Equal?(x=w296, y=20) -> (x >= y?=w297:bool)
          }
          n95 = while {
            shift-right: [w281] -> _
            shift-left: w252 -> [w288]
            shift-right: [w284] -> w243
            shift-left: w250 -> [w285]
            shift-right: [w282] -> w244
            shift-left: w248 -> [w282]
            tunnel: [w281] -> w242
            stop <- w287 stop-if-true
            n96 = call <vilib>:"WPI_EncoderGet.vi"("EncoderDevRef"=w285) -> ("Distance"=w286:dbl, "EncoderDevRef"=w284:T14)  [unwired: 5 in, 4 out]
            n97 = call-poly <vilib>:"WPI_RobotDriveArcadeDrive.vi"("Y axis value"=0.0 ("X axis value"), "X axis value"=0.5, "RobotDriveDevRef"=w288) -> ("RobotDriveDevRef"=w290:T6)  [unwired: 1 in, 7 out]
            n98 = Greater?(x=w286, y=120.0) -> (0:w287:bool)
            n99 = call <vilib>:"WPI_RobotDriveDelayAndUpdateSafety.vi"("Delay (s)"=0.05, "RobotDriveDevRef"=w290) -> ("RobotDriveDevRef 2"=w281:T6)  [unwired: 8 in, 1 out]
          }
          n100 = while {
            shift-right: [w275] -> w245
            shift-left: w244 -> [w274]
            shift-right: [w273] -> w246
            shift-left: w243 -> [w273]
            shift-right: [w272] -> w247
            shift-left: w242 -> [w272]
            i -> [w279]
            stop <- w280 stop-if-true
            n101 = Wait (ms)(milliseconds to wait=u32 50) -> ()  [unwired: 1 out]
            n102 = call-poly <vilib>:"WPI_SolenoidSet.vi"("Value"=WPI_SolenoidValue."Off", "SolenoidDevRef"=w274) -> ("SolenoidDevRef"=w275:T4)  [unwired: 8 in, 1 out]
            n103 = Greater Or Equal?(x=w279, y=20) -> (x >= y?=w280:bool)
          }
          n104 = while {
            tunnel: [w265] -> w260
            tunnel: w247 -> [w264]
            tunnel: w246 -> [w263]
            tunnel: [w262] -> w259
            tunnel: w245 -> [w261]
            tunnel: [w261] -> w258
            stop <- w271 stop-if-true
            (unwired) 0.5 ("X axis value")
            n105 = call <vilib>:"WPI_EncoderGet.vi"("EncoderDevRef"=w263) -> ("Distance"=w270:dbl, "EncoderDevRef"=w262:T14)  [unwired: 5 in, 4 out]
            n106 = call-poly <vilib>:"WPI_RobotDriveArcadeDrive.vi"("Y axis value"=0.0 ("X axis value"), "RobotDriveDevRef"=w264) -> ("RobotDriveDevRef"=w267:T6)  [unwired: 2 in, 7 out]
            n107 = Greater Or Equal?(x=w270, y=24.0) -> (x >= y?=w271:bool)
            n108 = call <vilib>:"WPI_RobotDriveDelayAndUpdateSafety.vi"("Delay (s)"=0.05, "RobotDriveDevRef"=w267) -> ("RobotDriveDevRef 2"=w265:T6)  [unwired: 8 in, 1 out]
          }
          n109 = while {
            shift-right: [w320] -> w257
            shift-left: w260 -> [w323]
            shift-right: [w318] -> w249
            shift-left: w258 -> [w318]
            shift-right: [w317] -> _
            shift-left: w259 -> [w319]
            shift-right: [w316] -> w256
            shift-left: w239 -> [w316]
            stop <- w326 stop-if-true
            n110 = call <vilib>:"WPI_EncoderGet.vi"("EncoderDevRef"=w319) -> ("Distance"=w327:dbl, "EncoderDevRef"=w317:T14)  [unwired: 5 in, 4 out]
            n111 = call-poly <vilib>:"WPI_RobotDriveArcadeDrive.vi"("Y axis value"=0.5 ("X axis value"), "X axis value"=0.0, "RobotDriveDevRef"=w323) -> ("RobotDriveDevRef"=w322:T6)  [unwired: 1 in, 7 out]
            n112 = Greater?(x=w327, y=135.0) -> (0:w326:bool)
            n113 = call <vilib>:"WPI_RobotDriveDelayAndUpdateSafety.vi"("Delay (s)"=0.05, "RobotDriveDevRef"=w322) -> ("RobotDriveDevRef 2"=w320:T6)  [unwired: 8 in, 1 out]
          }
          n114 = while {
            shift-right: [w309] -> _
            shift-left: w257 -> [w313]
            shift-right: [w303] -> _
            shift-left: w249 -> [w304]
            shift-right: [w305] -> w238
            shift-left: w256 -> [w305]
            i -> [w308]
            stop <- w306 stop-if-true
            (unwired) 0.0 ("Set Start Time (s)")
            n115 = call-poly <vilib>:"WPI_RobotDriveArcadeDrive.vi"("Y axis value"=0.0, "X axis value"=0.0, "RobotDriveDevRef"=w313) -> ("RobotDriveDevRef"=w310:T6)  [unwired: 1 in, 7 out]
            n116 = call-poly <vilib>:"WPI_SolenoidSet.vi"("Value"=WPI_SolenoidValue."Off", "SolenoidDevRef"=w304) -> ("SolenoidDevRef"=w303:T4)  [unwired: 8 in, 1 out]
            n117 = call <vilib>:"WPI_RobotDriveDelayAndUpdateSafety.vi"("Delay (s)"=0.05, "RobotDriveDevRef"=w310) -> ("RobotDriveDevRef 2"=w309:T6)  [unwired: 8 in, 1 out]
            n118 = Equal?(x=w308, y=39) -> (x = y?=w306:bool)
          }
        }
        frame "4" {
          n119 = call <vilib>:"WPI_RobotDriveRefNum Registry Get.vi"("refnum name"="Left and Right Motors") -> ("RobotDriveDevRef"=w341:T6)  [unwired: 1 in, 9 out]
          n120 = call <vilib>:"WPI_EncoderRefNum Registry Get.vi"("refnum name"="DriveControlR") -> ("EncoderDevRef"=w339:T14)  [unwired: 9 in, 1 out]
          n121 = call <vilib>:"WPI_SolenoidRefNum Registry Get.vi"("refnum name"="Intake Piston") -> ("error out"=w338:errorcluster, "SolenoidDevRef"=w337:T4)  [unwired: 9 in]
          n122 = while {
            tunnel: w338 -> [w397]
            tunnel: [w397] -> _
            shift-right: [w393] -> w344
            shift-left: w337 -> [w394]
            shift-right: [w396] -> w342
            shift-left: w339 -> [w396]
            shift-right: [w388] -> w340
            shift-left: w341 -> [w388]
            i -> [w391]
            stop <- w392 stop-if-true
            n123 = Wait (ms)(milliseconds to wait=u32 50) -> ()  [unwired: 1 out]
            n124 = call-poly <vilib>:"WPI_SolenoidSet.vi"("Value"=WPI_SolenoidValue."On", "SolenoidDevRef"=w394) -> ("SolenoidDevRef"=w393:T4)  [unwired: 8 in, 1 out]
            n125 = Greater Or Equal?(x=w391, y=20) -> (x >= y?=w392:bool)
          }
          n126 = while {
            shift-right: [w376] -> _
            shift-left: w340 -> [w383]
            shift-right: [w379] -> w349
            shift-left: w342 -> [w380]
            shift-right: [w377] -> w348
            shift-left: w344 -> [w377]
            tunnel: [w376] -> w350
            stop <- w382 stop-if-true
            n127 = call <vilib>:"WPI_EncoderGet.vi"("EncoderDevRef"=w380) -> ("Distance"=w381:dbl, "EncoderDevRef"=w379:T14)  [unwired: 5 in, 4 out]
            n128 = call-poly <vilib>:"WPI_RobotDriveArcadeDrive.vi"("Y axis value"=0.0 ("X axis value"), "X axis value"=0.5, "RobotDriveDevRef"=w383) -> ("RobotDriveDevRef"=w385:T6)  [unwired: 1 in, 7 out]
            n129 = Greater?(x=w381, y=120.0) -> (0:w382:bool)
            n130 = call <vilib>:"WPI_RobotDriveDelayAndUpdateSafety.vi"("Delay (s)"=0.05, "RobotDriveDevRef"=w385) -> ("RobotDriveDevRef 2"=w376:T6)  [unwired: 8 in, 1 out]
          }
          n131 = while {
            shift-right: [w370] -> w347
            shift-left: w348 -> [w369]
            shift-right: [w368] -> w346
            shift-left: w349 -> [w368]
            shift-right: [w367] -> w345
            shift-left: w350 -> [w367]
            i -> [w374]
            stop <- w375 stop-if-true
            n132 = Wait (ms)(milliseconds to wait=u32 50) -> ()  [unwired: 1 out]
            n133 = call-poly <vilib>:"WPI_SolenoidSet.vi"("Value"=WPI_SolenoidValue."Off", "SolenoidDevRef"=w369) -> ("SolenoidDevRef"=w370:T4)  [unwired: 8 in, 1 out]
            n134 = Greater Or Equal?(x=w374, y=20) -> (x >= y?=w375:bool)
          }
          n135 = while {
            tunnel: [w360] -> w351
            tunnel: w345 -> [w359]
            tunnel: w346 -> [w358]
            tunnel: [w357] -> w352
            tunnel: w347 -> [w356]
            tunnel: [w356] -> w353
            stop <- w366 stop-if-true
            (unwired) 0.5 ("X axis value")
            n136 = call <vilib>:"WPI_EncoderGet.vi"("EncoderDevRef"=w358) -> ("Distance"=w365:dbl, "EncoderDevRef"=w357:T14)  [unwired: 5 in, 4 out]
            n137 = call-poly <vilib>:"WPI_RobotDriveArcadeDrive.vi"("Y axis value"=0.0 ("X axis value"), "RobotDriveDevRef"=w359) -> ("RobotDriveDevRef"=w362:T6)  [unwired: 2 in, 7 out]
            n138 = Greater Or Equal?(x=w365, y=24.0) -> (x >= y?=w366:bool)
            n139 = call <vilib>:"WPI_RobotDriveDelayAndUpdateSafety.vi"("Delay (s)"=0.05, "RobotDriveDevRef"=w362) -> ("RobotDriveDevRef 2"=w360:T6)  [unwired: 8 in, 1 out]
          }
          n140 = while {
            shift-right: [w436] -> w332
            shift-left: w351 -> [w428]
            shift-right: [w424] -> w334
            shift-left: w353 -> [w425]
            shift-right: [w427] -> w333
            shift-left: w352 -> [w429]
            stop <- w430 stop-if-true
            n141 = call <vilib>:"WPI_EncoderGet.vi"("EncoderDevRef"=w429) -> ("Distance"=w431:dbl, "EncoderDevRef"=w427:T14)  [unwired: 5 in, 4 out]
            n142 = call-poly <vilib>:"WPI_RobotDriveArcadeDrive.vi"("Y axis value"=0.0 ("X axis value"), "X axis value"=0.5, "RobotDriveDevRef"=w428) -> ("RobotDriveDevRef"=w435:T6)  [unwired: 1 in, 7 out]
            n143 = Greater?(x=w431, y=-3.0) -> (0:w430:bool)
            n144 = call-poly <vilib>:"WPI_SolenoidSet.vi"("Value"=WPI_SolenoidValue."On", "SolenoidDevRef"=w425) -> ("SolenoidDevRef"=w424:T4)  [unwired: 8 in, 1 out]
            n145 = call <vilib>:"WPI_RobotDriveDelayAndUpdateSafety.vi"("Delay (s)"=0.05, "RobotDriveDevRef"=w435) -> ("RobotDriveDevRef 2"=w436:T6)  [unwired: 8 in, 1 out]
          }
          n146 = while {
            shift-right: [w415] -> w335
            shift-left: w332 -> [w418]
            shift-right: [w413] -> w343
            shift-left: w334 -> [w413]
            shift-right: [w412] -> _
            shift-left: w333 -> [w414]
            shift-right: [w411] -> w336
            shift-left: w330 -> [w411]
            stop <- w421 stop-if-true
            n147 = call <vilib>:"WPI_EncoderGet.vi"("EncoderDevRef"=w414) -> ("Distance"=w422:dbl, "EncoderDevRef"=w412:T14)  [unwired: 5 in, 4 out]
            n148 = call-poly <vilib>:"WPI_RobotDriveArcadeDrive.vi"("Y axis value"=0.5 ("X axis value"), "X axis value"=0.0, "RobotDriveDevRef"=w418) -> ("RobotDriveDevRef"=w417:T6)  [unwired: 1 in, 7 out]
            n149 = Greater?(x=w422, y=135.0) -> (0:w421:bool)
            n150 = call <vilib>:"WPI_RobotDriveDelayAndUpdateSafety.vi"("Delay (s)"=0.05, "RobotDriveDevRef"=w417) -> ("RobotDriveDevRef 2"=w415:T6)  [unwired: 8 in, 1 out]
          }
          n151 = while {
            shift-right: [w404] -> _
            shift-left: w335 -> [w408]
            shift-right: [w398] -> _
            shift-left: w343 -> [w399]
            shift-right: [w400] -> w331
            shift-left: w336 -> [w400]
            i -> [w403]
            stop <- w401 stop-if-true
            (unwired) 0.0 ("Set Start Time (s)")
            n152 = call-poly <vilib>:"WPI_RobotDriveArcadeDrive.vi"("Y axis value"=0.0, "X axis value"=0.0, "RobotDriveDevRef"=w408) -> ("RobotDriveDevRef"=w405:T6)  [unwired: 1 in, 7 out]
            n153 = call-poly <vilib>:"WPI_SolenoidSet.vi"("Value"=WPI_SolenoidValue."Off", "SolenoidDevRef"=w399) -> ("SolenoidDevRef"=w398:T4)  [unwired: 8 in, 1 out]
            n154 = call <vilib>:"WPI_RobotDriveDelayAndUpdateSafety.vi"("Delay (s)"=0.05, "RobotDriveDevRef"=w405) -> ("RobotDriveDevRef 2"=w404:T6)  [unwired: 8 in, 1 out]
            n155 = Equal?(x=w403, y=39) -> (x = y?=w401:bool)
          }
        }
        frame "5" {
          n156 = call <vilib>:"WPI_RobotDriveRefNum Registry Get.vi"("refnum name"="Left and Right Motors") -> ("RobotDriveDevRef"=w455:T6)  [unwired: 1 in, 9 out]
          n157 = call <vilib>:"WPI_EncoderRefNum Registry Get.vi"("refnum name"="DriveControlR") -> ("EncoderDevRef"=w457:T14)  [unwired: 9 in, 1 out]
          n158 = call <vilib>:"WPI_SolenoidRefNum Registry Get.vi"("refnum name"="Intake Piston") -> ("error out"=w458:errorcluster, "SolenoidDevRef"=w459:T4)  [unwired: 9 in]
          n159 = while {
            tunnel: w458 -> [w506]
            tunnel: [w506] -> _
            shift-right: [w502] -> w452
            shift-left: w459 -> [w503]
            shift-right: [w505] -> w454
            shift-left: w457 -> [w505]
            shift-right: [w497] -> w456
            shift-left: w455 -> [w497]
            i -> [w500]
            stop <- w501 stop-if-true
            n160 = Wait (ms)(milliseconds to wait=u32 50) -> ()  [unwired: 1 out]
            n161 = call-poly <vilib>:"WPI_SolenoidSet.vi"("Value"=WPI_SolenoidValue."On", "SolenoidDevRef"=w503) -> ("SolenoidDevRef"=w502:T4)  [unwired: 8 in, 1 out]
            n162 = Greater Or Equal?(x=w500, y=20) -> (x >= y?=w501:bool)
          }
          n163 = while {
            shift-right: [w485] -> _
            shift-left: w456 -> [w492]
            shift-right: [w488] -> w447
            shift-left: w454 -> [w489]
            shift-right: [w486] -> w448
            shift-left: w452 -> [w486]
            tunnel: [w485] -> w446
            stop <- w491 stop-if-true
            n164 = call <vilib>:"WPI_EncoderGet.vi"("EncoderDevRef"=w489) -> ("Distance"=w490:dbl, "EncoderDevRef"=w488:T14)  [unwired: 5 in, 4 out]
            n165 = call-poly <vilib>:"WPI_RobotDriveArcadeDrive.vi"("Y axis value"=0.0 ("X axis value"), "X axis value"=0.5, "RobotDriveDevRef"=w492) -> ("RobotDriveDevRef"=w494:T6)  [unwired: 1 in, 7 out]
            n166 = Greater?(x=w490, y=120.0) -> (0:w491:bool)
            n167 = call <vilib>:"WPI_RobotDriveDelayAndUpdateSafety.vi"("Delay (s)"=0.05, "RobotDriveDevRef"=w494) -> ("RobotDriveDevRef 2"=w485:T6)  [unwired: 8 in, 1 out]
          }
          n168 = while {
            shift-right: [w479] -> w449
            shift-left: w448 -> [w478]
            shift-right: [w477] -> w450
            shift-left: w447 -> [w477]
            shift-right: [w476] -> w451
            shift-left: w446 -> [w476]
            i -> [w483]
            stop <- w484 stop-if-true
            n169 = Wait (ms)(milliseconds to wait=u32 50) -> ()  [unwired: 1 out]
            n170 = call-poly <vilib>:"WPI_SolenoidSet.vi"("Value"=WPI_SolenoidValue."Off", "SolenoidDevRef"=w478) -> ("SolenoidDevRef"=w479:T4)  [unwired: 8 in, 1 out]
            n171 = Greater Or Equal?(x=w483, y=20) -> (x >= y?=w484:bool)
          }
          n172 = while {
            tunnel: [w469] -> w445
            tunnel: w451 -> [w468]
            tunnel: w450 -> [w467]
            tunnel: [w466] -> w444
            tunnel: w449 -> [w465]
            tunnel: [w465] -> w443
            stop <- w475 stop-if-true
            (unwired) 0.5 ("X axis value")
            n173 = call <vilib>:"WPI_EncoderGet.vi"("EncoderDevRef"=w467) -> ("Distance"=w474:dbl, "EncoderDevRef"=w466:T14)  [unwired: 5 in, 4 out]
            n174 = call-poly <vilib>:"WPI_RobotDriveArcadeDrive.vi"("Y axis value"=0.0 ("X axis value"), "RobotDriveDevRef"=w468) -> ("RobotDriveDevRef"=w471:T6)  [unwired: 2 in, 7 out]
            n175 = Greater Or Equal?(x=w474, y=24.0) -> (x >= y?=w475:bool)
            n176 = call <vilib>:"WPI_RobotDriveDelayAndUpdateSafety.vi"("Delay (s)"=0.05, "RobotDriveDevRef"=w471) -> ("RobotDriveDevRef 2"=w469:T6)  [unwired: 8 in, 1 out]
          }
          n177 = while {
            shift-right: [w545] -> w464
            shift-left: w445 -> [w537]
            shift-right: [w533] -> w462
            shift-left: w443 -> [w534]
            shift-right: [w536] -> w463
            shift-left: w444 -> [w538]
            stop <- w539 stop-if-true
            n178 = call <vilib>:"WPI_EncoderGet.vi"("EncoderDevRef"=w538) -> ("Distance"=w540:dbl, "EncoderDevRef"=w536:T14)  [unwired: 5 in, 4 out]
            n179 = call-poly <vilib>:"WPI_RobotDriveArcadeDrive.vi"("Y axis value"=0.0 ("X axis value"), "X axis value"=0.5, "RobotDriveDevRef"=w537) -> ("RobotDriveDevRef"=w544:T6)  [unwired: 1 in, 7 out]
            n180 = Greater?(x=w540, y=-6.0) -> (0:w539:bool)
            n181 = call-poly <vilib>:"WPI_SolenoidSet.vi"("Value"=WPI_SolenoidValue."On", "SolenoidDevRef"=w534) -> ("SolenoidDevRef"=w533:T4)  [unwired: 8 in, 1 out]
            n182 = call <vilib>:"WPI_RobotDriveDelayAndUpdateSafety.vi"("Delay (s)"=0.05, "RobotDriveDevRef"=w544) -> ("RobotDriveDevRef 2"=w545:T6)  [unwired: 8 in, 1 out]
          }
          n183 = while {
            shift-right: [w524] -> w461
            shift-left: w464 -> [w527]
            shift-right: [w522] -> w453
            shift-left: w462 -> [w522]
            shift-right: [w521] -> _
            shift-left: w463 -> [w523]
            shift-right: [w520] -> w460
            shift-left: w440 -> [w520]
            stop <- w530 stop-if-true
            n184 = call <vilib>:"WPI_EncoderGet.vi"("EncoderDevRef"=w523) -> ("Distance"=w531:dbl, "EncoderDevRef"=w521:T14)  [unwired: 5 in, 4 out]
            n185 = call-poly <vilib>:"WPI_RobotDriveArcadeDrive.vi"("Y axis value"=0.5 ("X axis value"), "X axis value"=0.0, "RobotDriveDevRef"=w527) -> ("RobotDriveDevRef"=w526:T6)  [unwired: 1 in, 7 out]
            n186 = Greater?(x=w531, y=135.0) -> (0:w530:bool)
            n187 = call <vilib>:"WPI_RobotDriveDelayAndUpdateSafety.vi"("Delay (s)"=0.05, "RobotDriveDevRef"=w526) -> ("RobotDriveDevRef 2"=w524:T6)  [unwired: 8 in, 1 out]
          }
          n188 = while {
            shift-right: [w513] -> _
            shift-left: w461 -> [w517]
            shift-right: [w507] -> _
            shift-left: w453 -> [w508]
            shift-right: [w509] -> w439
            shift-left: w460 -> [w509]
            i -> [w512]
            stop <- w510 stop-if-true
            (unwired) 0.0 ("Set Start Time (s)")
            n189 = call-poly <vilib>:"WPI_RobotDriveArcadeDrive.vi"("Y axis value"=0.0, "X axis value"=0.0, "RobotDriveDevRef"=w517) -> ("RobotDriveDevRef"=w514:T6)  [unwired: 1 in, 7 out]
            n190 = call-poly <vilib>:"WPI_SolenoidSet.vi"("Value"=WPI_SolenoidValue."Off", "SolenoidDevRef"=w508) -> ("SolenoidDevRef"=w507:T4)  [unwired: 8 in, 1 out]
            n191 = call <vilib>:"WPI_RobotDriveDelayAndUpdateSafety.vi"("Delay (s)"=0.05, "RobotDriveDevRef"=w514) -> ("RobotDriveDevRef 2"=w513:T6)  [unwired: 8 in, 1 out]
            n192 = Equal?(x=w512, y=39) -> (x = y?=w510:bool)
          }
        }
      }
      n193 = while {
        shift-right: [w553] -> w17
        shift-left: w14 -> [w558]
        i -> [w556]
        stop <- w554 stop-if-true
        n194 = call-poly <vilib>:"WPI_SolenoidSet.vi"("Value"=WPI_SolenoidValue."On", "SolenoidDevRef"=w558) -> ("SolenoidDevRef"=w553:T4)  [unwired: 8 in, 1 out]
        n195 = Greater Or Equal?(x=w556, y=39) -> (x >= y?=w554:bool)
      }
      n196 = while {
        shift-right: [w547] -> _
        shift-left: w17 -> [w552]
        i -> [w550]
        stop <- w548 stop-if-true
        n197 = call-poly <vilib>:"WPI_SolenoidSet.vi"("Value"=WPI_SolenoidValue."Off", "SolenoidDevRef"=w552) -> ("SolenoidDevRef"=w547:T4)  [unwired: 8 in, 1 out]
        n198 = Greater Or Equal?(x=w550, y=39) -> (x >= y?=w548:bool)
      }
    }
    frame "Rock Wall" {
      n199 = call <vilib>:"WPI_SolenoidRefNum Registry Get.vi"("refnum name"="Launch") -> ("SolenoidDevRef"=w560:T4)  [unwired: 9 in, 1 out]
      n200 = case shown="\"1\", Default" w559 {
        tunnel: [w564 w638 w714 w769 w843] -> w561
        tunnel: w560 -> [w565 w637 w713 w768 w841]
        frame "1", Default {
          n201 = call <vilib>:"WPI_SolenoidRefNum Registry Get.vi"("refnum name"="Intake Piston") -> ("error out"=w574:errorcluster, "SolenoidDevRef"=w575:T4)  [unwired: 9 in]
          n202 = call <vilib>:"WPI_EncoderRefNum Registry Get.vi"("refnum name"="DriveControlR") -> ("error out"=w578:errorcluster, "EncoderDevRef"=w579:T14)  [unwired: 9 in]
          n203 = call <vilib>:"WPI_RobotDriveRefNum Registry Get.vi"("refnum name"="Left and Right Motors") -> ("RobotDriveDevRef"=w582:T6)  [unwired: 1 in, 9 out]
          n204 = while {
            shift-right: [w634] -> w580
            shift-left: w582 -> [w636]
            tunnel: w578 -> [w626]
            tunnel: w575 -> [w624]
            tunnel: w574 -> [w623]
            shift-right: [w622] -> w573
            shift-left: _ -> [_]
            shift-right: [w625] -> w576
            shift-left: w579 -> [w627]
            stop <- w630 stop-if-true
            n205 = call <vilib>:"WPI_EncoderGet.vi"("error in (no error)"=w626, "EncoderDevRef"=w627) -> ("Distance"=w629:dbl, "EncoderDevRef"=w625:T14)  [unwired: 4 in, 4 out]
            n206 = call-poly <vilib>:"WPI_RobotDriveArcadeDrive.vi"("Y axis value"=0.5 ("X axis value"), "X axis value"=0.0, "RobotDriveDevRef"=w636) -> ("RobotDriveDevRef"=w633:T6)  [unwired: 1 in, 7 out]
            n207 = call-poly <vilib>:"WPI_SolenoidSet.vi"("error in (no error)"=w623, "Value"=WPI_SolenoidValue."On", "SolenoidDevRef"=w624) -> ("SolenoidDevRef"=w622:T4)  [unwired: 7 in, 1 out]
            n208 = Greater?(x=w629, y=248.0) -> (0:w630:bool)
            n209 = call <vilib>:"WPI_RobotDriveDelayAndUpdateSafety.vi"("Delay (s)"=0.05, "RobotDriveDevRef"=w633) -> ("RobotDriveDevRef 2"=w634:T6)  [unwired: 8 in, 1 out]
          }
          n210 = while {
            shift-right: [w619] -> w571
            shift-left: w580 -> [w611]
            shift-right: [w609] -> w568
            shift-left: w573 -> [w609]
            shift-right: [w610] -> w570
            shift-left: w576 -> [w612]
            stop <- w613 stop-if-true
            n211 = call <vilib>:"WPI_EncoderGet.vi"("EncoderDevRef"=w612) -> ("Distance"=w614:dbl, "EncoderDevRef"=w610:T14)  [unwired: 5 in, 4 out]
            n212 = call-poly <vilib>:"WPI_RobotDriveArcadeDrive.vi"("Y axis value"=0.0 ("X axis value"), "X axis value"=0.5, "RobotDriveDevRef"=w611) -> ("RobotDriveDevRef"=w618:T6)  [unwired: 1 in, 7 out]
            n213 = Greater?(x=w614, y=6.0) -> (0:w613:bool)
            n214 = call <vilib>:"WPI_RobotDriveDelayAndUpdateSafety.vi"("Delay (s)"=0.05, "RobotDriveDevRef"=w618) -> ("RobotDriveDevRef 2"=w619:T6)  [unwired: 8 in, 1 out]
          }
          n215 = while {
            shift-right: [w600] -> w567
            shift-left: w571 -> [w603]
            shift-right: [w598] -> w569
            shift-left: w568 -> [w598]
            shift-right: [w597] -> _
            shift-left: w570 -> [w599]
            shift-right: [w596] -> w566
            shift-left: w565 -> [w596]
            stop <- w606 stop-if-true
            n216 = call <vilib>:"WPI_EncoderGet.vi"("EncoderDevRef"=w599) -> ("Distance"=w607:dbl, "EncoderDevRef"=w597:T14)  [unwired: 5 in, 4 out]
            n217 = call-poly <vilib>:"WPI_RobotDriveArcadeDrive.vi"("Y axis value"=0.5 ("X axis value"), "X axis value"=0.0, "RobotDriveDevRef"=w603) -> ("RobotDriveDevRef"=w602:T6)  [unwired: 1 in, 7 out]
            n218 = Greater?(x=w607, y=135.0) -> (0:w606:bool)
            n219 = call <vilib>:"WPI_RobotDriveDelayAndUpdateSafety.vi"("Delay (s)"=0.05, "RobotDriveDevRef"=w602) -> ("RobotDriveDevRef 2"=w600:T6)  [unwired: 8 in, 1 out]
          }
          n220 = while {
            shift-right: [w588] -> _
            shift-left: w567 -> [w592]
            shift-right: [w587] -> _
            shift-left: w569 -> [w594]
            shift-right: [w583] -> w564
            shift-left: w566 -> [w583]
            i -> [w586]
            stop <- w584 stop-if-true
            (unwired) 0.0 ("Set Start Time (s)")
            n221 = call-poly <vilib>:"WPI_RobotDriveArcadeDrive.vi"("Y axis value"=0.0, "X axis value"=0.0, "RobotDriveDevRef"=w592) -> ("RobotDriveDevRef"=w589:T6)  [unwired: 1 in, 7 out]
            n222 = call-poly <vilib>:"WPI_SolenoidSet.vi"("Value"=WPI_SolenoidValue."Off", "SolenoidDevRef"=w594) -> ("SolenoidDevRef"=w587:T4)  [unwired: 8 in, 1 out]
            n223 = call <vilib>:"WPI_RobotDriveDelayAndUpdateSafety.vi"("Delay (s)"=0.05, "RobotDriveDevRef"=w589) -> ("RobotDriveDevRef 2"=w588:T6)  [unwired: 8 in, 1 out]
            n224 = Equal?(x=w586, y=39) -> (x = y?=w584:bool)
          }
        }
        frame "2" {
          n225 = call <vilib>:"WPI_SolenoidRefNum Registry Get.vi"("refnum name"="Intake Piston") -> ("error out"=w647:errorcluster, "SolenoidDevRef"=w648:T4)  [unwired: 9 in]
          n226 = call <vilib>:"WPI_EncoderRefNum Registry Get.vi"("refnum name"="DriveControlR") -> ("error out"=w651:errorcluster, "EncoderDevRef"=w652:T14)  [unwired: 9 in]
          n227 = call <vilib>:"WPI_RobotDriveRefNum Registry Get.vi"("refnum name"="Left and Right Motors") -> ("RobotDriveDevRef"=w655:T6)  [unwired: 1 in, 9 out]
          n228 = while {
            shift-right: [w707] -> w653
            shift-left: w655 -> [w709]
            tunnel: w651 -> [w699]
            tunnel: w648 -> [w697]
            tunnel: w647 -> [w696]
            shift-right: [w695] -> w646
            shift-left: _ -> [_]
            shift-right: [w698] -> w649
            shift-left: w652 -> [w700]
            stop <- w703 stop-if-true
            n229 = call <vilib>:"WPI_EncoderGet.vi"("error in (no error)"=w699, "EncoderDevRef"=w700) -> ("Distance"=w702:dbl, "EncoderDevRef"=w698:T14)  [unwired: 4 in, 4 out]
            n230 = call-poly <vilib>:"WPI_RobotDriveArcadeDrive.vi"("Y axis value"=0.5 ("X axis value"), "X axis value"=0.0, "RobotDriveDevRef"=w709) -> ("RobotDriveDevRef"=w706:T6)  [unwired: 1 in, 7 out]
            n231 = call-poly <vilib>:"WPI_SolenoidSet.vi"("error in (no error)"=w696, "Value"=WPI_SolenoidValue."On", "SolenoidDevRef"=w697) -> ("SolenoidDevRef"=w695:T4)  [unwired: 7 in, 1 out]
            n232 = Greater?(x=w702, y=248.0) -> (0:w703:bool)
            n233 = call <vilib>:"WPI_RobotDriveDelayAndUpdateSafety.vi"("Delay (s)"=0.05, "RobotDriveDevRef"=w706) -> ("RobotDriveDevRef 2"=w707:T6)  [unwired: 8 in, 1 out]
          }
          n234 = while {
            shift-right: [w692] -> w644
            shift-left: w653 -> [w684]
            shift-right: [w682] -> w641
            shift-left: w646 -> [w682]
            shift-right: [w683] -> w643
            shift-left: w649 -> [w685]
            stop <- w686 stop-if-true
            n235 = call <vilib>:"WPI_EncoderGet.vi"("EncoderDevRef"=w685) -> ("Distance"=w687:dbl, "EncoderDevRef"=w683:T14)  [unwired: 5 in, 4 out]
            n236 = call-poly <vilib>:"WPI_RobotDriveArcadeDrive.vi"("Y axis value"=0.0 ("X axis value"), "X axis value"=0.5, "RobotDriveDevRef"=w684) -> ("RobotDriveDevRef"=w691:T6)  [unwired: 1 in, 7 out]
            n237 = Greater?(x=w687, y=3.0) -> (0:w686:bool)
            n238 = call <vilib>:"WPI_RobotDriveDelayAndUpdateSafety.vi"("Delay (s)"=0.05, "RobotDriveDevRef"=w691) -> ("RobotDriveDevRef 2"=w692:T6)  [unwired: 8 in, 1 out]
          }
          n239 = while {
            shift-right: [w673] -> w640
            shift-left: w644 -> [w676]
            shift-right: [w671] -> w642
            shift-left: w641 -> [w671]
            shift-right: [w670] -> _
            shift-left: w643 -> [w672]
            shift-right: [w669] -> w639
            shift-left: w637 -> [w669]
            stop <- w679 stop-if-true
            n240 = call <vilib>:"WPI_EncoderGet.vi"("EncoderDevRef"=w672) -> ("Distance"=w680:dbl, "EncoderDevRef"=w670:T14)  [unwired: 5 in, 4 out]
            n241 = call-poly <vilib>:"WPI_RobotDriveArcadeDrive.vi"("Y axis value"=0.5 ("X axis value"), "X axis value"=0.0, "RobotDriveDevRef"=w676) -> ("RobotDriveDevRef"=w675:T6)  [unwired: 1 in, 7 out]
            n242 = Greater?(x=w680, y=135.0) -> (0:w679:bool)
            n243 = call <vilib>:"WPI_RobotDriveDelayAndUpdateSafety.vi"("Delay (s)"=0.05, "RobotDriveDevRef"=w675) -> ("RobotDriveDevRef 2"=w673:T6)  [unwired: 8 in, 1 out]
          }
          n244 = while {
            shift-right: [w661] -> _
            shift-left: w640 -> [w665]
            shift-right: [w660] -> _
            shift-left: w642 -> [w667]
            shift-right: [w656] -> w638
            shift-left: w639 -> [w656]
            i -> [w659]
            stop <- w657 stop-if-true
            (unwired) 0.0 ("Set Start Time (s)")
            n245 = call-poly <vilib>:"WPI_RobotDriveArcadeDrive.vi"("Y axis value"=0.0, "X axis value"=0.0, "RobotDriveDevRef"=w665) -> ("RobotDriveDevRef"=w662:T6)  [unwired: 1 in, 7 out]
            n246 = call-poly <vilib>:"WPI_SolenoidSet.vi"("Value"=WPI_SolenoidValue."Off", "SolenoidDevRef"=w667) -> ("SolenoidDevRef"=w660:T4)  [unwired: 8 in, 1 out]
            n247 = call <vilib>:"WPI_RobotDriveDelayAndUpdateSafety.vi"("Delay (s)"=0.05, "RobotDriveDevRef"=w662) -> ("RobotDriveDevRef 2"=w661:T6)  [unwired: 8 in, 1 out]
            n248 = Equal?(x=w659, y=39) -> (x = y?=w657:bool)
          }
        }
        frame "3" {
          n249 = call <vilib>:"WPI_SolenoidRefNum Registry Get.vi"("refnum name"="Intake Piston") -> ("error out"=w719:errorcluster, "SolenoidDevRef"=w720:T4)  [unwired: 9 in]
          n250 = call <vilib>:"WPI_EncoderRefNum Registry Get.vi"("refnum name"="DriveControlR") -> ("error out"=w722:errorcluster, "EncoderDevRef"=w723:T14)  [unwired: 9 in]
          n251 = call <vilib>:"WPI_RobotDriveRefNum Registry Get.vi"("refnum name"="Left and Right Motors") -> ("RobotDriveDevRef"=w725:T6)  [unwired: 1 in, 9 out]
          n252 = while {
            shift-right: [w765] -> w710
            shift-left: w725 -> [w767]
            tunnel: w722 -> [w757]
            tunnel: w720 -> [w755]
            tunnel: w719 -> [w754]
            shift-right: [w753] -> w712
            shift-left: _ -> [_]
            shift-right: [w756] -> w711
            shift-left: w723 -> [w758]
            stop <- w761 stop-if-true
            n253 = call <vilib>:"WPI_EncoderGet.vi"("error in (no error)"=w757, "EncoderDevRef"=w758) -> ("Distance"=w760:dbl, "EncoderDevRef"=w756:T14)  [unwired: 4 in, 4 out]
            n254 = call-poly <vilib>:"WPI_RobotDriveArcadeDrive.vi"("Y axis value"=0.5 ("X axis value"), "X axis value"=0.0, "RobotDriveDevRef"=w767) -> ("RobotDriveDevRef"=w764:T6)  [unwired: 1 in, 7 out]
            n255 = call-poly <vilib>:"WPI_SolenoidSet.vi"("error in (no error)"=w754, "Value"=WPI_SolenoidValue."On", "SolenoidDevRef"=w755) -> ("SolenoidDevRef"=w753:T4)  [unwired: 7 in, 1 out]
            n256 = Greater?(x=w760, y=248.0) -> (0:w761:bool)
            n257 = call <vilib>:"WPI_RobotDriveDelayAndUpdateSafety.vi"("Delay (s)"=0.05, "RobotDriveDevRef"=w764) -> ("RobotDriveDevRef 2"=w765:T6)  [unwired: 8 in, 1 out]
          }
          n258 = while {
            shift-right: [w743] -> w716
            shift-left: w710 -> [w746]
            shift-right: [w741] -> w717
            shift-left: w712 -> [w741]
            shift-right: [w740] -> _
            shift-left: w711 -> [w742]
            shift-right: [w739] -> w715
            shift-left: w713 -> [w739]
            stop <- w749 stop-if-true
            n259 = call <vilib>:"WPI_EncoderGet.vi"("EncoderDevRef"=w742) -> ("Distance"=w750:dbl, "EncoderDevRef"=w740:T14)  [unwired: 5 in, 4 out]
            n260 = call-poly <vilib>:"WPI_RobotDriveArcadeDrive.vi"("Y axis value"=0.5 ("X axis value"), "X axis value"=0.0, "RobotDriveDevRef"=w746) -> ("RobotDriveDevRef"=w745:T6)  [unwired: 1 in, 7 out]
            n261 = Greater?(x=w750, y=135.0) -> (0:w749:bool)
            n262 = call <vilib>:"WPI_RobotDriveDelayAndUpdateSafety.vi"("Delay (s)"=0.05, "RobotDriveDevRef"=w745) -> ("RobotDriveDevRef 2"=w743:T6)  [unwired: 8 in, 1 out]
          }
          n263 = while {
            shift-right: [w731] -> _
            shift-left: w716 -> [w735]
            shift-right: [w730] -> _
            shift-left: w717 -> [w737]
            shift-right: [w726] -> w714
            shift-left: w715 -> [w726]
            i -> [w729]
            stop <- w727 stop-if-true
            (unwired) 0.0 ("Set Start Time (s)")
            n264 = call-poly <vilib>:"WPI_RobotDriveArcadeDrive.vi"("Y axis value"=0.0, "X axis value"=0.0, "RobotDriveDevRef"=w735) -> ("RobotDriveDevRef"=w732:T6)  [unwired: 1 in, 7 out]
            n265 = call-poly <vilib>:"WPI_SolenoidSet.vi"("Value"=WPI_SolenoidValue."Off", "SolenoidDevRef"=w737) -> ("SolenoidDevRef"=w730:T4)  [unwired: 8 in, 1 out]
            n266 = call <vilib>:"WPI_RobotDriveDelayAndUpdateSafety.vi"("Delay (s)"=0.05, "RobotDriveDevRef"=w732) -> ("RobotDriveDevRef 2"=w731:T6)  [unwired: 8 in, 1 out]
            n267 = Equal?(x=w729, y=39) -> (x = y?=w727:bool)
          }
        }
        frame "4" {
          n268 = call <vilib>:"WPI_SolenoidRefNum Registry Get.vi"("refnum name"="Intake Piston") -> ("error out"=w778:errorcluster, "SolenoidDevRef"=w779:T4)  [unwired: 9 in]
          n269 = call <vilib>:"WPI_EncoderRefNum Registry Get.vi"("refnum name"="DriveControlR") -> ("error out"=w782:errorcluster, "EncoderDevRef"=w783:T14)  [unwired: 9 in]
          n270 = call <vilib>:"WPI_RobotDriveRefNum Registry Get.vi"("refnum name"="Left and Right Motors") -> ("RobotDriveDevRef"=w786:T6)  [unwired: 1 in, 9 out]
          n271 = while {
            shift-right: [w838] -> w784
            shift-left: w786 -> [w840]
            tunnel: w782 -> [w830]
            tunnel: w779 -> [w828]
            tunnel: w778 -> [w827]
            shift-right: [w826] -> w777
            shift-left: _ -> [_]
            shift-right: [w829] -> w780
            shift-left: w783 -> [w831]
            stop <- w834 stop-if-true
            n272 = call <vilib>:"WPI_EncoderGet.vi"("error in (no error)"=w830, "EncoderDevRef"=w831) -> ("Distance"=w833:dbl, "EncoderDevRef"=w829:T14)  [unwired: 4 in, 4 out]
            n273 = call-poly <vilib>:"WPI_RobotDriveArcadeDrive.vi"("Y axis value"=0.5 ("X axis value"), "X axis value"=0.0, "RobotDriveDevRef"=w840) -> ("RobotDriveDevRef"=w837:T6)  [unwired: 1 in, 7 out]
            n274 = call-poly <vilib>:"WPI_SolenoidSet.vi"("error in (no error)"=w827, "Value"=WPI_SolenoidValue."On", "SolenoidDevRef"=w828) -> ("SolenoidDevRef"=w826:T4)  [unwired: 7 in, 1 out]
            n275 = Greater?(x=w833, y=248.0) -> (0:w834:bool)
            n276 = call <vilib>:"WPI_RobotDriveDelayAndUpdateSafety.vi"("Delay (s)"=0.05, "RobotDriveDevRef"=w837) -> ("RobotDriveDevRef 2"=w838:T6)  [unwired: 8 in, 1 out]
          }
          n277 = while {
            shift-right: [w823] -> w775
            shift-left: w784 -> [w815]
            shift-right: [w813] -> w772
            shift-left: w777 -> [w813]
            shift-right: [w814] -> w774
            shift-left: w780 -> [w816]
            stop <- w817 stop-if-true
            n278 = call <vilib>:"WPI_EncoderGet.vi"("EncoderDevRef"=w816) -> ("Distance"=w818:dbl, "EncoderDevRef"=w814:T14)  [unwired: 5 in, 4 out]
            n279 = call-poly <vilib>:"WPI_RobotDriveArcadeDrive.vi"("Y axis value"=0.0 ("X axis value"), "X axis value"=0.5, "RobotDriveDevRef"=w815) -> ("RobotDriveDevRef"=w822:T6)  [unwired: 1 in, 7 out]
            n280 = Greater?(x=w818, y=-3.0) -> (0:w817:bool)
            n281 = call <vilib>:"WPI_RobotDriveDelayAndUpdateSafety.vi"("Delay (s)"=0.05, "RobotDriveDevRef"=w822) -> ("RobotDriveDevRef 2"=w823:T6)  [unwired: 8 in, 1 out]
          }
          n282 = while {
            shift-right: [w804] -> w771
            shift-left: w775 -> [w807]
            shift-right: [w802] -> w773
            shift-left: w772 -> [w802]
            shift-right: [w801] -> _
            shift-left: w774 -> [w803]
            shift-right: [w800] -> w770
            shift-left: w768 -> [w800]
            stop <- w810 stop-if-true
            n283 = call <vilib>:"WPI_EncoderGet.vi"("EncoderDevRef"=w803) -> ("Distance"=w811:dbl, "EncoderDevRef"=w801:T14)  [unwired: 5 in, 4 out]
            n284 = call-poly <vilib>:"WPI_RobotDriveArcadeDrive.vi"("Y axis value"=0.5 ("X axis value"), "X axis value"=0.0, "RobotDriveDevRef"=w807) -> ("RobotDriveDevRef"=w806:T6)  [unwired: 1 in, 7 out]
            n285 = Greater?(x=w811, y=135.0) -> (0:w810:bool)
            n286 = call <vilib>:"WPI_RobotDriveDelayAndUpdateSafety.vi"("Delay (s)"=0.05, "RobotDriveDevRef"=w806) -> ("RobotDriveDevRef 2"=w804:T6)  [unwired: 8 in, 1 out]
          }
          n287 = while {
            shift-right: [w792] -> _
            shift-left: w771 -> [w796]
            shift-right: [w791] -> _
            shift-left: w773 -> [w798]
            shift-right: [w787] -> w769
            shift-left: w770 -> [w787]
            i -> [w790]
            stop <- w788 stop-if-true
            (unwired) 0.0 ("Set Start Time (s)")
            n288 = call-poly <vilib>:"WPI_RobotDriveArcadeDrive.vi"("Y axis value"=0.0, "X axis value"=0.0, "RobotDriveDevRef"=w796) -> ("RobotDriveDevRef"=w793:T6)  [unwired: 1 in, 7 out]
            n289 = call-poly <vilib>:"WPI_SolenoidSet.vi"("Value"=WPI_SolenoidValue."Off", "SolenoidDevRef"=w798) -> ("SolenoidDevRef"=w791:T4)  [unwired: 8 in, 1 out]
            n290 = call <vilib>:"WPI_RobotDriveDelayAndUpdateSafety.vi"("Delay (s)"=0.05, "RobotDriveDevRef"=w793) -> ("RobotDriveDevRef 2"=w792:T6)  [unwired: 8 in, 1 out]
            n291 = Equal?(x=w790, y=39) -> (x = y?=w788:bool)
          }
        }
        frame "5" {
          n292 = call <vilib>:"WPI_SolenoidRefNum Registry Get.vi"("refnum name"="Intake Piston") -> ("error out"=w851:errorcluster, "SolenoidDevRef"=w852:T4)  [unwired: 9 in]
          n293 = call <vilib>:"WPI_EncoderRefNum Registry Get.vi"("refnum name"="DriveControlR") -> ("error out"=w855:errorcluster, "EncoderDevRef"=w856:T14)  [unwired: 9 in]
          n294 = call <vilib>:"WPI_RobotDriveRefNum Registry Get.vi"("refnum name"="Left and Right Motors") -> ("RobotDriveDevRef"=w859:T6)  [unwired: 1 in, 9 out]
          n295 = while {
            shift-right: [w911] -> w857
            shift-left: w859 -> [w913]
            tunnel: w855 -> [w903]
            tunnel: w852 -> [w901]
            tunnel: w851 -> [w900]
            shift-right: [w899] -> w850
            shift-left: _ -> [_]
            shift-right: [w902] -> w853
            shift-left: w856 -> [w904]
            stop <- w907 stop-if-true
            n296 = call <vilib>:"WPI_EncoderGet.vi"("error in (no error)"=w903, "EncoderDevRef"=w904) -> ("Distance"=w906:dbl, "EncoderDevRef"=w902:T14)  [unwired: 4 in, 4 out]
            n297 = call-poly <vilib>:"WPI_RobotDriveArcadeDrive.vi"("Y axis value"=0.5 ("X axis value"), "X axis value"=0.0, "RobotDriveDevRef"=w913) -> ("RobotDriveDevRef"=w910:T6)  [unwired: 1 in, 7 out]
            n298 = call-poly <vilib>:"WPI_SolenoidSet.vi"("error in (no error)"=w900, "Value"=WPI_SolenoidValue."On", "SolenoidDevRef"=w901) -> ("SolenoidDevRef"=w899:T4)  [unwired: 7 in, 1 out]
            n299 = Greater?(x=w906, y=248.0) -> (0:w907:bool)
            n300 = call <vilib>:"WPI_RobotDriveDelayAndUpdateSafety.vi"("Delay (s)"=0.05, "RobotDriveDevRef"=w910) -> ("RobotDriveDevRef 2"=w911:T6)  [unwired: 8 in, 1 out]
          }
          n301 = while {
            shift-right: [w896] -> w848
            shift-left: w857 -> [w888]
            shift-right: [w886] -> w845
            shift-left: w850 -> [w886]
            shift-right: [w887] -> w847
            shift-left: w853 -> [w889]
            stop <- w890 stop-if-true
            n302 = call <vilib>:"WPI_EncoderGet.vi"("EncoderDevRef"=w889) -> ("Distance"=w891:dbl, "EncoderDevRef"=w887:T14)  [unwired: 5 in, 4 out]
            n303 = call-poly <vilib>:"WPI_RobotDriveArcadeDrive.vi"("Y axis value"=0.0 ("X axis value"), "X axis value"=0.5, "RobotDriveDevRef"=w888) -> ("RobotDriveDevRef"=w895:T6)  [unwired: 1 in, 7 out]
            n304 = Greater?(x=w891, y=-6.0) -> (0:w890:bool)
            n305 = call <vilib>:"WPI_RobotDriveDelayAndUpdateSafety.vi"("Delay (s)"=0.05, "RobotDriveDevRef"=w895) -> ("RobotDriveDevRef 2"=w896:T6)  [unwired: 8 in, 1 out]
          }
          n306 = while {
            shift-right: [w877] -> w844
            shift-left: w848 -> [w880]
            shift-right: [w875] -> w846
            shift-left: w845 -> [w875]
            shift-right: [w874] -> _
            shift-left: w847 -> [w876]
            shift-right: [w873] -> w842
            shift-left: w841 -> [w873]
            stop <- w883 stop-if-true
            n307 = call <vilib>:"WPI_EncoderGet.vi"("EncoderDevRef"=w876) -> ("Distance"=w884:dbl, "EncoderDevRef"=w874:T14)  [unwired: 5 in, 4 out]
            n308 = call-poly <vilib>:"WPI_RobotDriveArcadeDrive.vi"("Y axis value"=0.5 ("X axis value"), "X axis value"=0.0, "RobotDriveDevRef"=w880) -> ("RobotDriveDevRef"=w879:T6)  [unwired: 1 in, 7 out]
            n309 = Greater?(x=w884, y=135.0) -> (0:w883:bool)
            n310 = call <vilib>:"WPI_RobotDriveDelayAndUpdateSafety.vi"("Delay (s)"=0.05, "RobotDriveDevRef"=w879) -> ("RobotDriveDevRef 2"=w877:T6)  [unwired: 8 in, 1 out]
          }
          n311 = while {
            shift-right: [w865] -> _
            shift-left: w844 -> [w869]
            shift-right: [w864] -> _
            shift-left: w846 -> [w871]
            shift-right: [w860] -> w843
            shift-left: w842 -> [w860]
            i -> [w863]
            stop <- w861 stop-if-true
            (unwired) 0.0 ("Set Start Time (s)")
            n312 = call-poly <vilib>:"WPI_RobotDriveArcadeDrive.vi"("Y axis value"=0.0, "X axis value"=0.0, "RobotDriveDevRef"=w869) -> ("RobotDriveDevRef"=w866:T6)  [unwired: 1 in, 7 out]
            n313 = call-poly <vilib>:"WPI_SolenoidSet.vi"("Value"=WPI_SolenoidValue."Off", "SolenoidDevRef"=w871) -> ("SolenoidDevRef"=w864:T4)  [unwired: 8 in, 1 out]
            n314 = call <vilib>:"WPI_RobotDriveDelayAndUpdateSafety.vi"("Delay (s)"=0.05, "RobotDriveDevRef"=w866) -> ("RobotDriveDevRef 2"=w865:T6)  [unwired: 8 in, 1 out]
            n315 = Equal?(x=w863, y=39) -> (x = y?=w861:bool)
          }
        }
      }
      n316 = while {
        shift-right: [w920] -> w562
        shift-left: w561 -> [w925]
        i -> [w923]
        stop <- w921 stop-if-true
        n317 = call-poly <vilib>:"WPI_SolenoidSet.vi"("Value"=WPI_SolenoidValue."On", "SolenoidDevRef"=w925) -> ("SolenoidDevRef"=w920:T4)  [unwired: 8 in, 1 out]
        n318 = Greater Or Equal?(x=w923, y=39) -> (x >= y?=w921:bool)
      }
      n319 = while {
        shift-right: [w914] -> _
        shift-left: w562 -> [w919]
        i -> [w917]
        stop <- w915 stop-if-true
        n320 = call-poly <vilib>:"WPI_SolenoidSet.vi"("Value"=WPI_SolenoidValue."Off", "SolenoidDevRef"=w919) -> ("SolenoidDevRef"=w914:T4)  [unwired: 8 in, 1 out]
        n321 = Greater Or Equal?(x=w917, y=39) -> (x >= y?=w915:bool)
      }
    }
    frame "Lowbar", Default {
      # "Code for the lowbar. \n\n1. move forward 248 inches, raise pneumatic arm\n2. turn 6 inches\n3. move forward 135 inches\n4. drop pneumatic arm and wait 2 seconds for the ball to settle\n5. shoot the catapult\n6. drop the catapult and wait"
      n322 = call <vilib>:"WPI_SolenoidRefNum Registry Get.vi"("refnum name"="Intake Piston") -> ("error out"=w938:errorcluster, "SolenoidDevRef"=w939:T4)  [unwired: 9 in]
      n323 = call <vilib>:"WPI_EncoderRefNum Registry Get.vi"("refnum name"="DriveControlR") -> ("error out"=w942:errorcluster, "EncoderDevRef"=w943:T14)  [unwired: 9 in]
      n324 = call <vilib>:"WPI_RobotDriveRefNum Registry Get.vi"("refnum name"="Left and Right Motors") -> ("RobotDriveDevRef"=w946:T6)  [unwired: 1 in, 9 out]
      n325 = while {
        shift-right: [w1011] -> w944
        shift-left: w946 -> [w1013]
        tunnel: w942 -> [w1003]
        tunnel: w939 -> [w1001]
        tunnel: w938 -> [w1000]
        shift-right: [w999] -> w937
        shift-left: _ -> [_]
        shift-right: [w1002] -> w940
        shift-left: w943 -> [w1004]
        stop <- w1007 stop-if-true
        n326 = call <vilib>:"WPI_EncoderGet.vi"("error in (no error)"=w1003, "EncoderDevRef"=w1004) -> ("Distance"=w1006:dbl, "EncoderDevRef"=w1002:T14)  [unwired: 4 in, 4 out]
        n327 = call-poly <vilib>:"WPI_RobotDriveArcadeDrive.vi"("Y axis value"=0.5 ("X axis value"), "X axis value"=0.0, "RobotDriveDevRef"=w1013) -> ("RobotDriveDevRef"=w1010:T6)  [unwired: 1 in, 7 out]
        n328 = call-poly <vilib>:"WPI_SolenoidSet.vi"("error in (no error)"=w1000, "Value"=WPI_SolenoidValue."On", "SolenoidDevRef"=w1001) -> ("SolenoidDevRef"=w999:T4)  [unwired: 7 in, 1 out]
        n329 = Greater?(x=w1006, y=248.0) -> (0:w1007:bool)
        n330 = call <vilib>:"WPI_RobotDriveDelayAndUpdateSafety.vi"("Delay (s)"=0.05, "RobotDriveDevRef"=w1010) -> ("RobotDriveDevRef 2"=w1011:T6)  [unwired: 8 in, 1 out]
      }
      n331 = while {
        shift-right: [w996] -> w935
        shift-left: w944 -> [w988]
        shift-right: [w986] -> w932
        shift-left: w937 -> [w986]
        shift-right: [w987] -> w934
        shift-left: w940 -> [w989]
        stop <- w990 stop-if-true
        n332 = call <vilib>:"WPI_EncoderGet.vi"("EncoderDevRef"=w989) -> ("Distance"=w991:dbl, "EncoderDevRef"=w987:T14)  [unwired: 5 in, 4 out]
        n333 = call-poly <vilib>:"WPI_RobotDriveArcadeDrive.vi"("Y axis value"=0.0 ("X axis value"), "X axis value"=0.5, "RobotDriveDevRef"=w988) -> ("RobotDriveDevRef"=w995:T6)  [unwired: 1 in, 7 out]
        n334 = Greater?(x=w991, y=6.0) -> (0:w990:bool)
        n335 = call <vilib>:"WPI_RobotDriveDelayAndUpdateSafety.vi"("Delay (s)"=0.05, "RobotDriveDevRef"=w995) -> ("RobotDriveDevRef 2"=w996:T6)  [unwired: 8 in, 1 out]
      }
      n336 = call <vilib>:"WPI_SolenoidRefNum Registry Get.vi"("refnum name"="Launch") -> ("SolenoidDevRef"=w928:T4)  [unwired: 9 in, 1 out]
      n337 = while {
        shift-right: [w977] -> w931
        shift-left: w935 -> [w980]
        shift-right: [w975] -> w933
        shift-left: w932 -> [w975]
        shift-right: [w974] -> _
        shift-left: w934 -> [w976]
        shift-right: [w973] -> w926
        shift-left: w928 -> [w973]
        stop <- w983 stop-if-true
        n338 = call <vilib>:"WPI_EncoderGet.vi"("EncoderDevRef"=w976) -> ("Distance"=w984:dbl, "EncoderDevRef"=w974:T14)  [unwired: 5 in, 4 out]
        n339 = call-poly <vilib>:"WPI_RobotDriveArcadeDrive.vi"("Y axis value"=0.5 ("X axis value"), "X axis value"=0.0, "RobotDriveDevRef"=w980) -> ("RobotDriveDevRef"=w979:T6)  [unwired: 1 in, 7 out]
        n340 = Greater?(x=w984, y=135.0) -> (0:w983:bool)
        n341 = call <vilib>:"WPI_RobotDriveDelayAndUpdateSafety.vi"("Delay (s)"=0.05, "RobotDriveDevRef"=w979) -> ("RobotDriveDevRef 2"=w977:T6)  [unwired: 8 in, 1 out]
      }
      n342 = while {
        shift-right: [w965] -> _
        shift-left: w931 -> [w969]
        shift-right: [w964] -> _
        shift-left: w933 -> [w971]
        shift-right: [w960] -> w927
        shift-left: w926 -> [w960]
        i -> [w963]
        stop <- w961 stop-if-true
        (unwired) 0.0 ("Set Start Time (s)")
        n343 = call-poly <vilib>:"WPI_RobotDriveArcadeDrive.vi"("Y axis value"=0.0, "X axis value"=0.0, "RobotDriveDevRef"=w969) -> ("RobotDriveDevRef"=w966:T6)  [unwired: 1 in, 7 out]
        n344 = call-poly <vilib>:"WPI_SolenoidSet.vi"("Value"=WPI_SolenoidValue."Off", "SolenoidDevRef"=w971) -> ("SolenoidDevRef"=w964:T4)  [unwired: 8 in, 1 out]
        n345 = call <vilib>:"WPI_RobotDriveDelayAndUpdateSafety.vi"("Delay (s)"=0.05, "RobotDriveDevRef"=w966) -> ("RobotDriveDevRef 2"=w965:T6)  [unwired: 8 in, 1 out]
        n346 = Equal?(x=w963, y=39) -> (x = y?=w961:bool)
      }
      n347 = while {
        shift-right: [w954] -> w929
        shift-left: w927 -> [w959]
        i -> [w957]
        stop <- w955 stop-if-true
        n348 = Wait (ms)(milliseconds to wait=u32 1 ("millisecond timer value")) -> ()  [unwired: 1 out]
        n349 = call-poly <vilib>:"WPI_SolenoidSet.vi"("Value"=WPI_SolenoidValue."On", "SolenoidDevRef"=w959) -> ("SolenoidDevRef"=w954:T4)  [unwired: 8 in, 1 out]
        n350 = Greater Or Equal?(x=w957, y=39) -> (x >= y?=w955:bool)
      }
      n351 = while {
        shift-right: [w947] -> _
        shift-left: w929 -> [w952]
        i -> [w950]
        stop <- w948 stop-if-true
        n352 = call-poly <vilib>:"WPI_SolenoidSet.vi"("Value"=WPI_SolenoidValue."Off", "SolenoidDevRef"=w952) -> ("SolenoidDevRef"=w947:T4)  [unwired: 8 in, 1 out]
        n353 = Greater Or Equal?(x=w950, y=39) -> (x >= y?=w948:bool)
      }
    }
    frame "Nothing" {
      # "Does absolutely nothing. last resort or if asked for by allience."
    }
    frame "Approach" {
      n354 = call <vilib>:"WPI_EncoderRefNum Registry Get.vi"("refnum name"="DriveControlR") -> ("EncoderDevRef"=w1017:T14)  [unwired: 9 in, 1 out]
      n355 = call <vilib>:"WPI_RobotDriveRefNum Registry Get.vi"("refnum name"="Left and Right Motors") -> ("RobotDriveDevRef"=w1014:T6)  [unwired: 1 in, 9 out]
      n356 = while {
        tunnel: w1017 -> [w1020]
        tunnel: w1014 -> [w1019]
        stop <- w1018 stop-if-true
        n357 = call <vilib>:"WPI_EncoderGet.vi"("EncoderDevRef"=w1020) -> ("Distance"=w1025:dbl)  [unwired: 5 in, 5 out]
        n358 = call-poly <vilib>:"WPI_RobotDriveArcadeDrive.vi"("Y axis value"=0.0 ("X axis value"), "X axis value"=0.5, "RobotDriveDevRef"=w1019) -> ("RobotDriveDevRef"=w1023:T6)  [unwired: 1 in, 7 out]
        n359 = Greater?(x=w1025, y=120.0) -> (0:w1018:bool)
        n360 = call <vilib>:"WPI_RobotDriveDelayAndUpdateSafety.vi"("Delay (s)"=0.05, "RobotDriveDevRef"=w1023) -> ()  [unwired: 8 in, 2 out]
      }
    }
    frame "Rough Terrain/Ramp Parts" {
      n361 = call <vilib>:"WPI_SolenoidRefNum Registry Get.vi"("refnum name"="Launch") -> ("SolenoidDevRef"=w1028:T4)  [unwired: 9 in, 1 out]
      n362 = case shown="\"1\", Default" w1027 {
        tunnel: [w1032 w1106 w1182 w1237 w1311] -> w1029
        tunnel: w1028 -> [w1033 w1105 w1181 w1236 w1309]
        frame "1", Default {
          n363 = call <vilib>:"WPI_SolenoidRefNum Registry Get.vi"("refnum name"="Intake Piston") -> ("error out"=w1042:errorcluster, "SolenoidDevRef"=w1043:T4)  [unwired: 9 in]
          n364 = call <vilib>:"WPI_EncoderRefNum Registry Get.vi"("refnum name"="DriveControlR") -> ("error out"=w1046:errorcluster, "EncoderDevRef"=w1047:T14)  [unwired: 9 in]
          n365 = call <vilib>:"WPI_RobotDriveRefNum Registry Get.vi"("refnum name"="Left and Right Motors") -> ("RobotDriveDevRef"=w1050:T6)  [unwired: 1 in, 9 out]
          n366 = while {
            shift-right: [w1102] -> w1048
            shift-left: w1050 -> [w1104]
            tunnel: w1046 -> [w1094]
            tunnel: w1043 -> [w1092]
            tunnel: w1042 -> [w1091]
            shift-right: [w1090] -> w1041
            shift-left: _ -> [_]
            shift-right: [w1093] -> w1044
            shift-left: w1047 -> [w1095]
            stop <- w1098 stop-if-true
            n367 = call <vilib>:"WPI_EncoderGet.vi"("error in (no error)"=w1094, "EncoderDevRef"=w1095) -> ("Distance"=w1097:dbl, "EncoderDevRef"=w1093:T14)  [unwired: 4 in, 4 out]
            n368 = call-poly <vilib>:"WPI_RobotDriveArcadeDrive.vi"("Y axis value"=0.5 ("X axis value"), "X axis value"=0.0, "RobotDriveDevRef"=w1104) -> ("RobotDriveDevRef"=w1101:T6)  [unwired: 1 in, 7 out]
            n369 = call-poly <vilib>:"WPI_SolenoidSet.vi"("error in (no error)"=w1091, "Value"=WPI_SolenoidValue."On", "SolenoidDevRef"=w1092) -> ("SolenoidDevRef"=w1090:T4)  [unwired: 7 in, 1 out]
            n370 = Greater?(x=w1097, y=248.0) -> (0:w1098:bool)
            n371 = call <vilib>:"WPI_RobotDriveDelayAndUpdateSafety.vi"("Delay (s)"=0.05, "RobotDriveDevRef"=w1101) -> ("RobotDriveDevRef 2"=w1102:T6)  [unwired: 8 in, 1 out]
          }
          n372 = while {
            shift-right: [w1087] -> w1039
            shift-left: w1048 -> [w1079]
            shift-right: [w1077] -> w1036
            shift-left: w1041 -> [w1077]
            shift-right: [w1078] -> w1038
            shift-left: w1044 -> [w1080]
            stop <- w1081 stop-if-true
            n373 = call <vilib>:"WPI_EncoderGet.vi"("EncoderDevRef"=w1080) -> ("Distance"=w1082:dbl, "EncoderDevRef"=w1078:T14)  [unwired: 5 in, 4 out]
            n374 = call-poly <vilib>:"WPI_RobotDriveArcadeDrive.vi"("Y axis value"=0.0 ("X axis value"), "X axis value"=0.5, "RobotDriveDevRef"=w1079) -> ("RobotDriveDevRef"=w1086:T6)  [unwired: 1 in, 7 out]
            n375 = Greater?(x=w1082, y=6.0) -> (0:w1081:bool)
            n376 = call <vilib>:"WPI_RobotDriveDelayAndUpdateSafety.vi"("Delay (s)"=0.05, "RobotDriveDevRef"=w1086) -> ("RobotDriveDevRef 2"=w1087:T6)  [unwired: 8 in, 1 out]
          }
          n377 = while {
            shift-right: [w1068] -> w1035
            shift-left: w1039 -> [w1071]
            shift-right: [w1066] -> w1037
            shift-left: w1036 -> [w1066]
            shift-right: [w1065] -> _
            shift-left: w1038 -> [w1067]
            shift-right: [w1064] -> w1034
            shift-left: w1033 -> [w1064]
            stop <- w1074 stop-if-true
            n378 = call <vilib>:"WPI_EncoderGet.vi"("EncoderDevRef"=w1067) -> ("Distance"=w1075:dbl, "EncoderDevRef"=w1065:T14)  [unwired: 5 in, 4 out]
            n379 = call-poly <vilib>:"WPI_RobotDriveArcadeDrive.vi"("Y axis value"=0.5 ("X axis value"), "X axis value"=0.0, "RobotDriveDevRef"=w1071) -> ("RobotDriveDevRef"=w1070:T6)  [unwired: 1 in, 7 out]
            n380 = Greater?(x=w1075, y=135.0) -> (0:w1074:bool)
            n381 = call <vilib>:"WPI_RobotDriveDelayAndUpdateSafety.vi"("Delay (s)"=0.05, "RobotDriveDevRef"=w1070) -> ("RobotDriveDevRef 2"=w1068:T6)  [unwired: 8 in, 1 out]
          }
          n382 = while {
            shift-right: [w1056] -> _
            shift-left: w1035 -> [w1060]
            shift-right: [w1055] -> _
            shift-left: w1037 -> [w1062]
            shift-right: [w1051] -> w1032
            shift-left: w1034 -> [w1051]
            i -> [w1054]
            stop <- w1052 stop-if-true
            (unwired) 0.0 ("Set Start Time (s)")
            n383 = call-poly <vilib>:"WPI_RobotDriveArcadeDrive.vi"("Y axis value"=0.0, "X axis value"=0.0, "RobotDriveDevRef"=w1060) -> ("RobotDriveDevRef"=w1057:T6)  [unwired: 1 in, 7 out]
            n384 = call-poly <vilib>:"WPI_SolenoidSet.vi"("Value"=WPI_SolenoidValue."Off", "SolenoidDevRef"=w1062) -> ("SolenoidDevRef"=w1055:T4)  [unwired: 8 in, 1 out]
            n385 = call <vilib>:"WPI_RobotDriveDelayAndUpdateSafety.vi"("Delay (s)"=0.05, "RobotDriveDevRef"=w1057) -> ("RobotDriveDevRef 2"=w1056:T6)  [unwired: 8 in, 1 out]
            n386 = Equal?(x=w1054, y=39) -> (x = y?=w1052:bool)
          }
        }
        frame "2" {
          n387 = call <vilib>:"WPI_SolenoidRefNum Registry Get.vi"("refnum name"="Intake Piston") -> ("error out"=w1115:errorcluster, "SolenoidDevRef"=w1116:T4)  [unwired: 9 in]
          n388 = call <vilib>:"WPI_EncoderRefNum Registry Get.vi"("refnum name"="DriveControlR") -> ("error out"=w1119:errorcluster, "EncoderDevRef"=w1120:T14)  [unwired: 9 in]
          n389 = call <vilib>:"WPI_RobotDriveRefNum Registry Get.vi"("refnum name"="Left and Right Motors") -> ("RobotDriveDevRef"=w1123:T6)  [unwired: 1 in, 9 out]
          n390 = while {
            shift-right: [w1175] -> w1121
            shift-left: w1123 -> [w1177]
            tunnel: w1119 -> [w1167]
            tunnel: w1116 -> [w1165]
            tunnel: w1115 -> [w1164]
            shift-right: [w1163] -> w1114
            shift-left: _ -> [_]
            shift-right: [w1166] -> w1117
            shift-left: w1120 -> [w1168]
            stop <- w1171 stop-if-true
            n391 = call <vilib>:"WPI_EncoderGet.vi"("error in (no error)"=w1167, "EncoderDevRef"=w1168) -> ("Distance"=w1170:dbl, "EncoderDevRef"=w1166:T14)  [unwired: 4 in, 4 out]
            n392 = call-poly <vilib>:"WPI_RobotDriveArcadeDrive.vi"("Y axis value"=0.5 ("X axis value"), "X axis value"=0.0, "RobotDriveDevRef"=w1177) -> ("RobotDriveDevRef"=w1174:T6)  [unwired: 1 in, 7 out]
            n393 = call-poly <vilib>:"WPI_SolenoidSet.vi"("error in (no error)"=w1164, "Value"=WPI_SolenoidValue."On", "SolenoidDevRef"=w1165) -> ("SolenoidDevRef"=w1163:T4)  [unwired: 7 in, 1 out]
            n394 = Greater?(x=w1170, y=248.0) -> (0:w1171:bool)
            n395 = call <vilib>:"WPI_RobotDriveDelayAndUpdateSafety.vi"("Delay (s)"=0.05, "RobotDriveDevRef"=w1174) -> ("RobotDriveDevRef 2"=w1175:T6)  [unwired: 8 in, 1 out]
          }
          n396 = while {
            shift-right: [w1160] -> w1112
            shift-left: w1121 -> [w1152]
            shift-right: [w1150] -> w1109
            shift-left: w1114 -> [w1150]
            shift-right: [w1151] -> w1111
            shift-left: w1117 -> [w1153]
            stop <- w1154 stop-if-true
            n397 = call <vilib>:"WPI_EncoderGet.vi"("EncoderDevRef"=w1153) -> ("Distance"=w1155:dbl, "EncoderDevRef"=w1151:T14)  [unwired: 5 in, 4 out]
            n398 = call-poly <vilib>:"WPI_RobotDriveArcadeDrive.vi"("Y axis value"=0.0 ("X axis value"), "X axis value"=0.5, "RobotDriveDevRef"=w1152) -> ("RobotDriveDevRef"=w1159:T6)  [unwired: 1 in, 7 out]
            n399 = Greater?(x=w1155, y=3.0) -> (0:w1154:bool)
            n400 = call <vilib>:"WPI_RobotDriveDelayAndUpdateSafety.vi"("Delay (s)"=0.05, "RobotDriveDevRef"=w1159) -> ("RobotDriveDevRef 2"=w1160:T6)  [unwired: 8 in, 1 out]
          }
          n401 = while {
            shift-right: [w1141] -> w1108
            shift-left: w1112 -> [w1144]
            shift-right: [w1139] -> w1110
            shift-left: w1109 -> [w1139]
            shift-right: [w1138] -> _
            shift-left: w1111 -> [w1140]
            shift-right: [w1137] -> w1107
            shift-left: w1105 -> [w1137]
            stop <- w1147 stop-if-true
            n402 = call <vilib>:"WPI_EncoderGet.vi"("EncoderDevRef"=w1140) -> ("Distance"=w1148:dbl, "EncoderDevRef"=w1138:T14)  [unwired: 5 in, 4 out]
            n403 = call-poly <vilib>:"WPI_RobotDriveArcadeDrive.vi"("Y axis value"=0.5 ("X axis value"), "X axis value"=0.0, "RobotDriveDevRef"=w1144) -> ("RobotDriveDevRef"=w1143:T6)  [unwired: 1 in, 7 out]
            n404 = Greater?(x=w1148, y=135.0) -> (0:w1147:bool)
            n405 = call <vilib>:"WPI_RobotDriveDelayAndUpdateSafety.vi"("Delay (s)"=0.05, "RobotDriveDevRef"=w1143) -> ("RobotDriveDevRef 2"=w1141:T6)  [unwired: 8 in, 1 out]
          }
          n406 = while {
            shift-right: [w1129] -> _
            shift-left: w1108 -> [w1133]
            shift-right: [w1128] -> _
            shift-left: w1110 -> [w1135]
            shift-right: [w1124] -> w1106
            shift-left: w1107 -> [w1124]
            i -> [w1127]
            stop <- w1125 stop-if-true
            (unwired) 0.0 ("Set Start Time (s)")
            n407 = call-poly <vilib>:"WPI_RobotDriveArcadeDrive.vi"("Y axis value"=0.0, "X axis value"=0.0, "RobotDriveDevRef"=w1133) -> ("RobotDriveDevRef"=w1130:T6)  [unwired: 1 in, 7 out]
            n408 = call-poly <vilib>:"WPI_SolenoidSet.vi"("Value"=WPI_SolenoidValue."Off", "SolenoidDevRef"=w1135) -> ("SolenoidDevRef"=w1128:T4)  [unwired: 8 in, 1 out]
            n409 = call <vilib>:"WPI_RobotDriveDelayAndUpdateSafety.vi"("Delay (s)"=0.05, "RobotDriveDevRef"=w1130) -> ("RobotDriveDevRef 2"=w1129:T6)  [unwired: 8 in, 1 out]
            n410 = Equal?(x=w1127, y=39) -> (x = y?=w1125:bool)
          }
        }
        frame "3" {
          n411 = call <vilib>:"WPI_SolenoidRefNum Registry Get.vi"("refnum name"="Intake Piston") -> ("error out"=w1187:errorcluster, "SolenoidDevRef"=w1188:T4)  [unwired: 9 in]
          n412 = call <vilib>:"WPI_EncoderRefNum Registry Get.vi"("refnum name"="DriveControlR") -> ("error out"=w1190:errorcluster, "EncoderDevRef"=w1191:T14)  [unwired: 9 in]
          n413 = call <vilib>:"WPI_RobotDriveRefNum Registry Get.vi"("refnum name"="Left and Right Motors") -> ("RobotDriveDevRef"=w1193:T6)  [unwired: 1 in, 9 out]
          n414 = while {
            shift-right: [w1233] -> w1178
            shift-left: w1193 -> [w1235]
            tunnel: w1190 -> [w1225]
            tunnel: w1188 -> [w1223]
            tunnel: w1187 -> [w1222]
            shift-right: [w1221] -> w1180
            shift-left: _ -> [_]
            shift-right: [w1224] -> w1179
            shift-left: w1191 -> [w1226]
            stop <- w1229 stop-if-true
            n415 = call <vilib>:"WPI_EncoderGet.vi"("error in (no error)"=w1225, "EncoderDevRef"=w1226) -> ("Distance"=w1228:dbl, "EncoderDevRef"=w1224:T14)  [unwired: 4 in, 4 out]
            n416 = call-poly <vilib>:"WPI_RobotDriveArcadeDrive.vi"("Y axis value"=0.5 ("X axis value"), "X axis value"=0.0, "RobotDriveDevRef"=w1235) -> ("RobotDriveDevRef"=w1232:T6)  [unwired: 1 in, 7 out]
            n417 = call-poly <vilib>:"WPI_SolenoidSet.vi"("error in (no error)"=w1222, "Value"=WPI_SolenoidValue."On", "SolenoidDevRef"=w1223) -> ("SolenoidDevRef"=w1221:T4)  [unwired: 7 in, 1 out]
            n418 = Greater?(x=w1228, y=248.0) -> (0:w1229:bool)
            n419 = call <vilib>:"WPI_RobotDriveDelayAndUpdateSafety.vi"("Delay (s)"=0.05, "RobotDriveDevRef"=w1232) -> ("RobotDriveDevRef 2"=w1233:T6)  [unwired: 8 in, 1 out]
          }
          n420 = while {
            shift-right: [w1211] -> w1184
            shift-left: w1178 -> [w1214]
            shift-right: [w1209] -> w1185
            shift-left: w1180 -> [w1209]
            shift-right: [w1208] -> _
            shift-left: w1179 -> [w1210]
            shift-right: [w1207] -> w1183
            shift-left: w1181 -> [w1207]
            stop <- w1217 stop-if-true
            n421 = call <vilib>:"WPI_EncoderGet.vi"("EncoderDevRef"=w1210) -> ("Distance"=w1218:dbl, "EncoderDevRef"=w1208:T14)  [unwired: 5 in, 4 out]
            n422 = call-poly <vilib>:"WPI_RobotDriveArcadeDrive.vi"("Y axis value"=0.5 ("X axis value"), "X axis value"=0.0, "RobotDriveDevRef"=w1214) -> ("RobotDriveDevRef"=w1213:T6)  [unwired: 1 in, 7 out]
            n423 = Greater?(x=w1218, y=135.0) -> (0:w1217:bool)
            n424 = call <vilib>:"WPI_RobotDriveDelayAndUpdateSafety.vi"("Delay (s)"=0.05, "RobotDriveDevRef"=w1213) -> ("RobotDriveDevRef 2"=w1211:T6)  [unwired: 8 in, 1 out]
          }
          n425 = while {
            shift-right: [w1199] -> _
            shift-left: w1184 -> [w1203]
            shift-right: [w1198] -> _
            shift-left: w1185 -> [w1205]
            shift-right: [w1194] -> w1182
            shift-left: w1183 -> [w1194]
            i -> [w1197]
            stop <- w1195 stop-if-true
            (unwired) 0.0 ("Set Start Time (s)")
            n426 = call-poly <vilib>:"WPI_RobotDriveArcadeDrive.vi"("Y axis value"=0.0, "X axis value"=0.0, "RobotDriveDevRef"=w1203) -> ("RobotDriveDevRef"=w1200:T6)  [unwired: 1 in, 7 out]
            n427 = call-poly <vilib>:"WPI_SolenoidSet.vi"("Value"=WPI_SolenoidValue."Off", "SolenoidDevRef"=w1205) -> ("SolenoidDevRef"=w1198:T4)  [unwired: 8 in, 1 out]
            n428 = call <vilib>:"WPI_RobotDriveDelayAndUpdateSafety.vi"("Delay (s)"=0.05, "RobotDriveDevRef"=w1200) -> ("RobotDriveDevRef 2"=w1199:T6)  [unwired: 8 in, 1 out]
            n429 = Equal?(x=w1197, y=39) -> (x = y?=w1195:bool)
          }
        }
        frame "4" {
          n430 = call <vilib>:"WPI_SolenoidRefNum Registry Get.vi"("refnum name"="Intake Piston") -> ("error out"=w1246:errorcluster, "SolenoidDevRef"=w1247:T4)  [unwired: 9 in]
          n431 = call <vilib>:"WPI_EncoderRefNum Registry Get.vi"("refnum name"="DriveControlR") -> ("error out"=w1250:errorcluster, "EncoderDevRef"=w1251:T14)  [unwired: 9 in]
          n432 = call <vilib>:"WPI_RobotDriveRefNum Registry Get.vi"("refnum name"="Left and Right Motors") -> ("RobotDriveDevRef"=w1254:T6)  [unwired: 1 in, 9 out]
          n433 = while {
            shift-right: [w1306] -> w1252
            shift-left: w1254 -> [w1308]
            tunnel: w1250 -> [w1298]
            tunnel: w1247 -> [w1296]
            tunnel: w1246 -> [w1295]
            shift-right: [w1294] -> w1245
            shift-left: _ -> [_]
            shift-right: [w1297] -> w1248
            shift-left: w1251 -> [w1299]
            stop <- w1302 stop-if-true
            n434 = call <vilib>:"WPI_EncoderGet.vi"("error in (no error)"=w1298, "EncoderDevRef"=w1299) -> ("Distance"=w1301:dbl, "EncoderDevRef"=w1297:T14)  [unwired: 4 in, 4 out]
            n435 = call-poly <vilib>:"WPI_RobotDriveArcadeDrive.vi"("Y axis value"=0.5 ("X axis value"), "X axis value"=0.0, "RobotDriveDevRef"=w1308) -> ("RobotDriveDevRef"=w1305:T6)  [unwired: 1 in, 7 out]
            n436 = call-poly <vilib>:"WPI_SolenoidSet.vi"("error in (no error)"=w1295, "Value"=WPI_SolenoidValue."On", "SolenoidDevRef"=w1296) -> ("SolenoidDevRef"=w1294:T4)  [unwired: 7 in, 1 out]
            n437 = Greater?(x=w1301, y=248.0) -> (0:w1302:bool)
            n438 = call <vilib>:"WPI_RobotDriveDelayAndUpdateSafety.vi"("Delay (s)"=0.05, "RobotDriveDevRef"=w1305) -> ("RobotDriveDevRef 2"=w1306:T6)  [unwired: 8 in, 1 out]
          }
          n439 = while {
            shift-right: [w1291] -> w1243
            shift-left: w1252 -> [w1283]
            shift-right: [w1281] -> w1240
            shift-left: w1245 -> [w1281]
            shift-right: [w1282] -> w1242
            shift-left: w1248 -> [w1284]
            stop <- w1285 stop-if-true
            n440 = call <vilib>:"WPI_EncoderGet.vi"("EncoderDevRef"=w1284) -> ("Distance"=w1286:dbl, "EncoderDevRef"=w1282:T14)  [unwired: 5 in, 4 out]
            n441 = call-poly <vilib>:"WPI_RobotDriveArcadeDrive.vi"("Y axis value"=0.0 ("X axis value"), "X axis value"=0.5, "RobotDriveDevRef"=w1283) -> ("RobotDriveDevRef"=w1290:T6)  [unwired: 1 in, 7 out]
            n442 = Greater?(x=w1286, y=-3.0) -> (0:w1285:bool)
            n443 = call <vilib>:"WPI_RobotDriveDelayAndUpdateSafety.vi"("Delay (s)"=0.05, "RobotDriveDevRef"=w1290) -> ("RobotDriveDevRef 2"=w1291:T6)  [unwired: 8 in, 1 out]
          }
          n444 = while {
            shift-right: [w1272] -> w1239
            shift-left: w1243 -> [w1275]
            shift-right: [w1270] -> w1241
            shift-left: w1240 -> [w1270]
            shift-right: [w1269] -> _
            shift-left: w1242 -> [w1271]
            shift-right: [w1268] -> w1238
            shift-left: w1236 -> [w1268]
            stop <- w1278 stop-if-true
            n445 = call <vilib>:"WPI_EncoderGet.vi"("EncoderDevRef"=w1271) -> ("Distance"=w1279:dbl, "EncoderDevRef"=w1269:T14)  [unwired: 5 in, 4 out]
            n446 = call-poly <vilib>:"WPI_RobotDriveArcadeDrive.vi"("Y axis value"=0.5 ("X axis value"), "X axis value"=0.0, "RobotDriveDevRef"=w1275) -> ("RobotDriveDevRef"=w1274:T6)  [unwired: 1 in, 7 out]
            n447 = Greater?(x=w1279, y=135.0) -> (0:w1278:bool)
            n448 = call <vilib>:"WPI_RobotDriveDelayAndUpdateSafety.vi"("Delay (s)"=0.05, "RobotDriveDevRef"=w1274) -> ("RobotDriveDevRef 2"=w1272:T6)  [unwired: 8 in, 1 out]
          }
          n449 = while {
            shift-right: [w1260] -> _
            shift-left: w1239 -> [w1264]
            shift-right: [w1259] -> _
            shift-left: w1241 -> [w1266]
            shift-right: [w1255] -> w1237
            shift-left: w1238 -> [w1255]
            i -> [w1258]
            stop <- w1256 stop-if-true
            (unwired) 0.0 ("Set Start Time (s)")
            n450 = call-poly <vilib>:"WPI_RobotDriveArcadeDrive.vi"("Y axis value"=0.0, "X axis value"=0.0, "RobotDriveDevRef"=w1264) -> ("RobotDriveDevRef"=w1261:T6)  [unwired: 1 in, 7 out]
            n451 = call-poly <vilib>:"WPI_SolenoidSet.vi"("Value"=WPI_SolenoidValue."Off", "SolenoidDevRef"=w1266) -> ("SolenoidDevRef"=w1259:T4)  [unwired: 8 in, 1 out]
            n452 = call <vilib>:"WPI_RobotDriveDelayAndUpdateSafety.vi"("Delay (s)"=0.05, "RobotDriveDevRef"=w1261) -> ("RobotDriveDevRef 2"=w1260:T6)  [unwired: 8 in, 1 out]
            n453 = Equal?(x=w1258, y=39) -> (x = y?=w1256:bool)
          }
        }
        frame "5" {
          n454 = call <vilib>:"WPI_SolenoidRefNum Registry Get.vi"("refnum name"="Intake Piston") -> ("error out"=w1319:errorcluster, "SolenoidDevRef"=w1320:T4)  [unwired: 9 in]
          n455 = call <vilib>:"WPI_EncoderRefNum Registry Get.vi"("refnum name"="DriveControlR") -> ("error out"=w1323:errorcluster, "EncoderDevRef"=w1324:T14)  [unwired: 9 in]
          n456 = call <vilib>:"WPI_RobotDriveRefNum Registry Get.vi"("refnum name"="Left and Right Motors") -> ("RobotDriveDevRef"=w1327:T6)  [unwired: 1 in, 9 out]
          n457 = while {
            shift-right: [w1379] -> w1325
            shift-left: w1327 -> [w1381]
            tunnel: w1323 -> [w1371]
            tunnel: w1320 -> [w1369]
            tunnel: w1319 -> [w1368]
            shift-right: [w1367] -> w1318
            shift-left: _ -> [_]
            shift-right: [w1370] -> w1321
            shift-left: w1324 -> [w1372]
            stop <- w1375 stop-if-true
            n458 = call <vilib>:"WPI_EncoderGet.vi"("error in (no error)"=w1371, "EncoderDevRef"=w1372) -> ("Distance"=w1374:dbl, "EncoderDevRef"=w1370:T14)  [unwired: 4 in, 4 out]
            n459 = call-poly <vilib>:"WPI_RobotDriveArcadeDrive.vi"("Y axis value"=0.5 ("X axis value"), "X axis value"=0.0, "RobotDriveDevRef"=w1381) -> ("RobotDriveDevRef"=w1378:T6)  [unwired: 1 in, 7 out]
            n460 = call-poly <vilib>:"WPI_SolenoidSet.vi"("error in (no error)"=w1368, "Value"=WPI_SolenoidValue."On", "SolenoidDevRef"=w1369) -> ("SolenoidDevRef"=w1367:T4)  [unwired: 7 in, 1 out]
            n461 = Greater?(x=w1374, y=248.0) -> (0:w1375:bool)
            n462 = call <vilib>:"WPI_RobotDriveDelayAndUpdateSafety.vi"("Delay (s)"=0.05, "RobotDriveDevRef"=w1378) -> ("RobotDriveDevRef 2"=w1379:T6)  [unwired: 8 in, 1 out]
          }
          n463 = while {
            shift-right: [w1364] -> w1316
            shift-left: w1325 -> [w1356]
            shift-right: [w1354] -> w1313
            shift-left: w1318 -> [w1354]
            shift-right: [w1355] -> w1315
            shift-left: w1321 -> [w1357]
            stop <- w1358 stop-if-true
            n464 = call <vilib>:"WPI_EncoderGet.vi"("EncoderDevRef"=w1357) -> ("Distance"=w1359:dbl, "EncoderDevRef"=w1355:T14)  [unwired: 5 in, 4 out]
            n465 = call-poly <vilib>:"WPI_RobotDriveArcadeDrive.vi"("Y axis value"=0.0 ("X axis value"), "X axis value"=0.5, "RobotDriveDevRef"=w1356) -> ("RobotDriveDevRef"=w1363:T6)  [unwired: 1 in, 7 out]
            n466 = Greater?(x=w1359, y=-6.0) -> (0:w1358:bool)
            n467 = call <vilib>:"WPI_RobotDriveDelayAndUpdateSafety.vi"("Delay (s)"=0.05, "RobotDriveDevRef"=w1363) -> ("RobotDriveDevRef 2"=w1364:T6)  [unwired: 8 in, 1 out]
          }
          n468 = while {
            shift-right: [w1345] -> w1312
            shift-left: w1316 -> [w1348]
            shift-right: [w1343] -> w1314
            shift-left: w1313 -> [w1343]
            shift-right: [w1342] -> _
            shift-left: w1315 -> [w1344]
            shift-right: [w1341] -> w1310
            shift-left: w1309 -> [w1341]
            stop <- w1351 stop-if-true
            n469 = call <vilib>:"WPI_EncoderGet.vi"("EncoderDevRef"=w1344) -> ("Distance"=w1352:dbl, "EncoderDevRef"=w1342:T14)  [unwired: 5 in, 4 out]
            n470 = call-poly <vilib>:"WPI_RobotDriveArcadeDrive.vi"("Y axis value"=0.5 ("X axis value"), "X axis value"=0.0, "RobotDriveDevRef"=w1348) -> ("RobotDriveDevRef"=w1347:T6)  [unwired: 1 in, 7 out]
            n471 = Greater?(x=w1352, y=135.0) -> (0:w1351:bool)
            n472 = call <vilib>:"WPI_RobotDriveDelayAndUpdateSafety.vi"("Delay (s)"=0.05, "RobotDriveDevRef"=w1347) -> ("RobotDriveDevRef 2"=w1345:T6)  [unwired: 8 in, 1 out]
          }
          n473 = while {
            shift-right: [w1333] -> _
            shift-left: w1312 -> [w1337]
            shift-right: [w1332] -> _
            shift-left: w1314 -> [w1339]
            shift-right: [w1328] -> w1311
            shift-left: w1310 -> [w1328]
            i -> [w1331]
            stop <- w1329 stop-if-true
            (unwired) 0.0 ("Set Start Time (s)")
            n474 = call-poly <vilib>:"WPI_RobotDriveArcadeDrive.vi"("Y axis value"=0.0, "X axis value"=0.0, "RobotDriveDevRef"=w1337) -> ("RobotDriveDevRef"=w1334:T6)  [unwired: 1 in, 7 out]
            n475 = call-poly <vilib>:"WPI_SolenoidSet.vi"("Value"=WPI_SolenoidValue."Off", "SolenoidDevRef"=w1339) -> ("SolenoidDevRef"=w1332:T4)  [unwired: 8 in, 1 out]
            n476 = call <vilib>:"WPI_RobotDriveDelayAndUpdateSafety.vi"("Delay (s)"=0.05, "RobotDriveDevRef"=w1334) -> ("RobotDriveDevRef 2"=w1333:T6)  [unwired: 8 in, 1 out]
            n477 = Equal?(x=w1331, y=39) -> (x = y?=w1329:bool)
          }
        }
      }
      n478 = while {
        shift-right: [w1388] -> w1030
        shift-left: w1029 -> [w1393]
        i -> [w1391]
        stop <- w1389 stop-if-true
        n479 = call-poly <vilib>:"WPI_SolenoidSet.vi"("Value"=WPI_SolenoidValue."On", "SolenoidDevRef"=w1393) -> ("SolenoidDevRef"=w1388:T4)  [unwired: 8 in, 1 out]
        n480 = Greater Or Equal?(x=w1391, y=39) -> (x >= y?=w1389:bool)
      }
      n481 = while {
        shift-right: [w1382] -> _
        shift-left: w1030 -> [w1387]
        i -> [w1385]
        stop <- w1383 stop-if-true
        n482 = call-poly <vilib>:"WPI_SolenoidSet.vi"("Value"=WPI_SolenoidValue."Off", "SolenoidDevRef"=w1387) -> ("SolenoidDevRef"=w1382:T4)  [unwired: 8 in, 1 out]
        n483 = Greater Or Equal?(x=w1385, y=39) -> (x >= y?=w1383:bool)
      }
    }
  }
